vi "Autonomous Independent.vi"   [LabVIEW 2017]
doc: "This VI is called when autonomous begins, and will automatically be terminated when autonomous ends. You can carry out timed or sensor driven robot movement independently without needing to return to the caller."
uses:
  AutonActions.ctl
  WristPositions.ctl
  fec7e146-7db9-40ed-95e9-9a867f74a6f6.vi
  cf8db7aa-b0ae-4ba0-9a67-042f718c3c26.vi
  <vilib>/Rock Robotics/Network Tables/NT Write String.vi
types:
  T1 = cluster{"TrgtCounts":i32, "CurrCounts":dbl, "SlowRng":dbl}
  T2 = cluster{"Heading":dbl, "Target":dbl, "Range":dbl, "GyroSens":dbl}
  T3 = typedef "AutonActions.ctl" = enum16{"Initialize", "Stop", "StraightForward", "StraightBack", "SolenoidControl", "StraightForwardTime", "Release", "Shoot", "Wrist", "GripperToggle", "ElevUp", "ElevDown", "Pause", "ShifterToggle", "", "CubeCollect", "Intake", "ForwardPivot", "BackPivot", "GeneralTurn"}
  T4 = typedef "WristPositions.ctl" = enum16{"AllDown", "AllUp"}
  T5 = cluster{"Action":T3, "DriveEncCnts":i32, "Accel?":bool, "Decel?":bool, "ElevEncCnts":i32, "Action2":T3, "Action2Trigger":i32, "WristPositions":T4, "SlowRng":dbl, "TimeOut":dbl, "GyroSens":dbl, "DriveHeading":dbl}[]
  T6 = cluster{"Action":T3, "DriveEncCnts":i32, "Accel?":bool, "Decel?":bool, "ElevEncCnts":i32, "Action2":T3, "Action2Trigger":i32, "WristPositions":T4, "SlowRng":dbl, "TimeOut":dbl, "GyroSens":dbl, "DriveHeading":dbl}
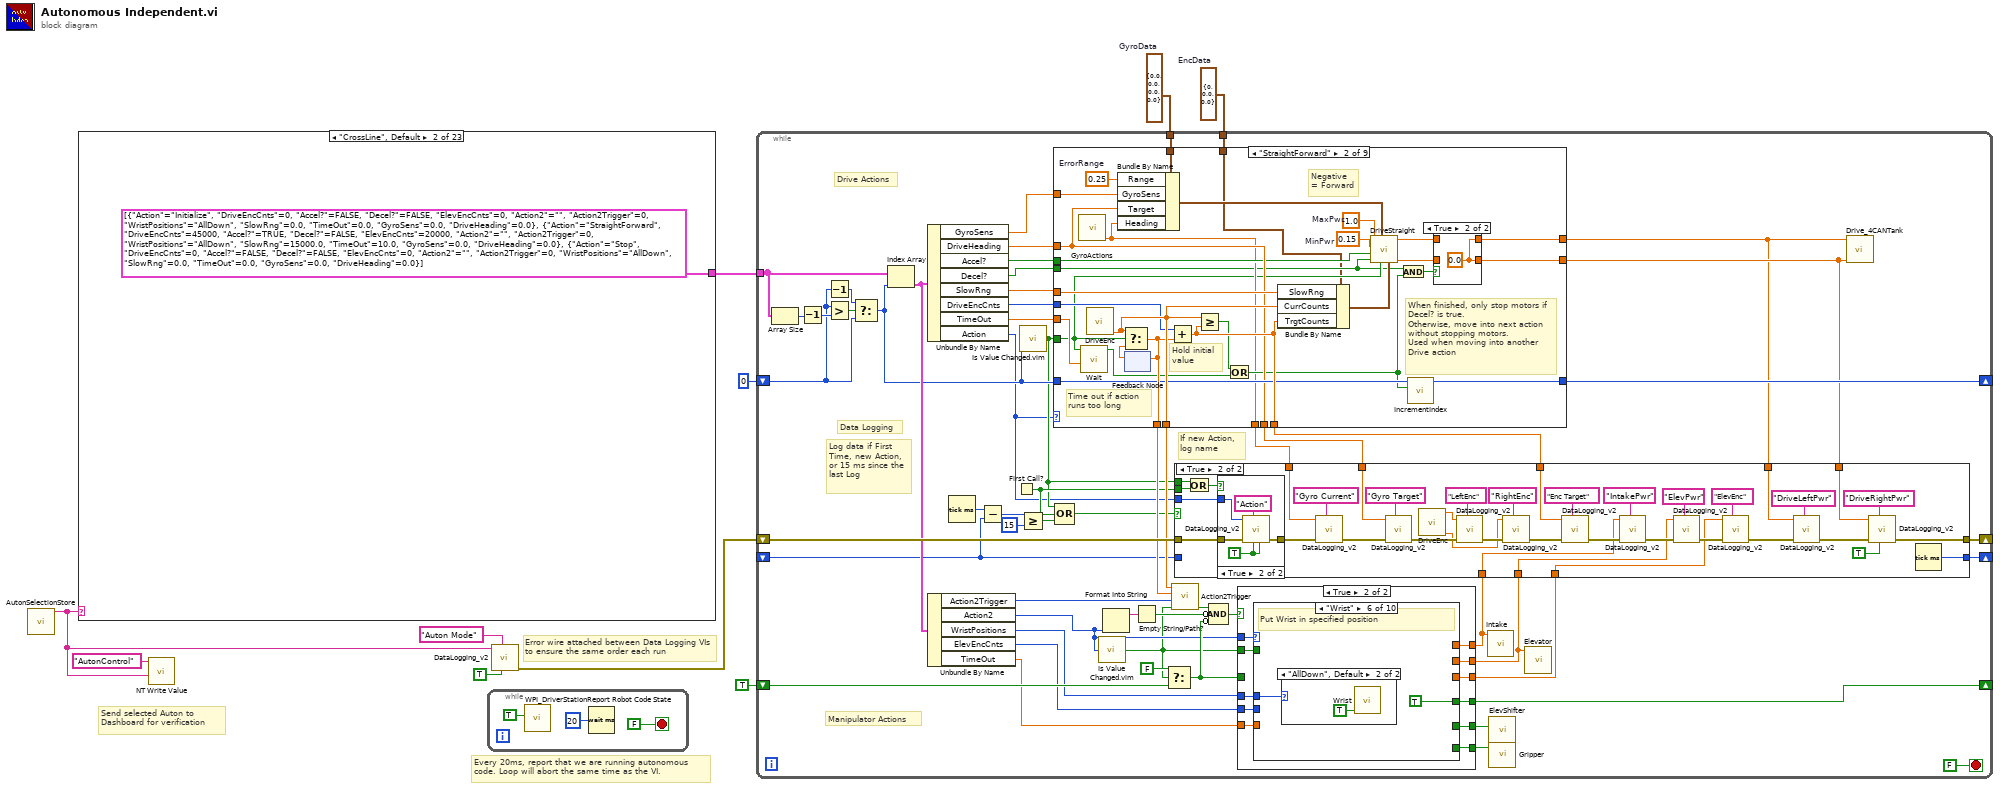
[diagram p0: block diagram]
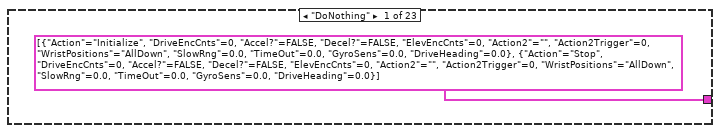
[diagram p2: hidden frame]
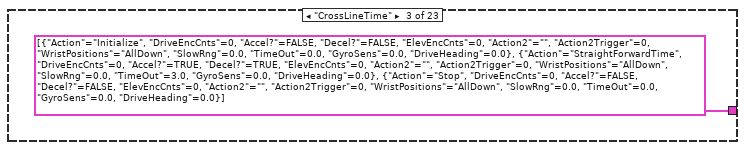
[diagram p3: hidden frame]
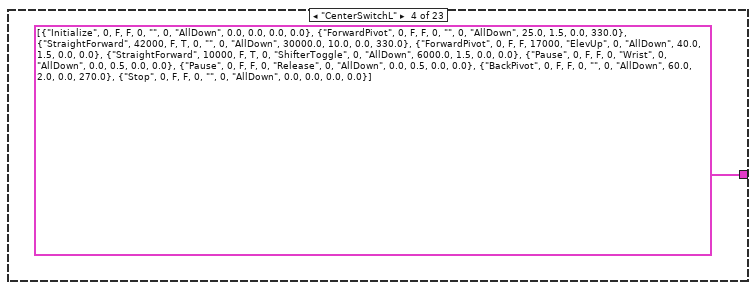
[diagram p4: hidden frame]
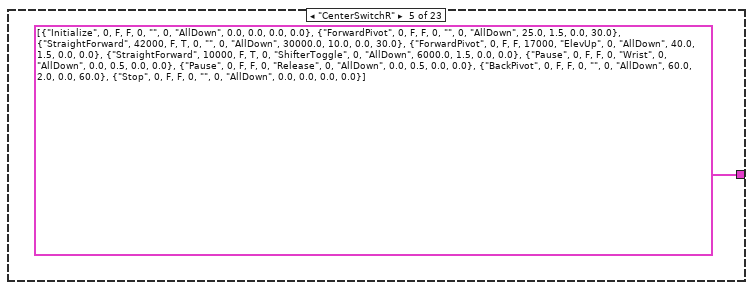
[diagram p5: hidden frame]
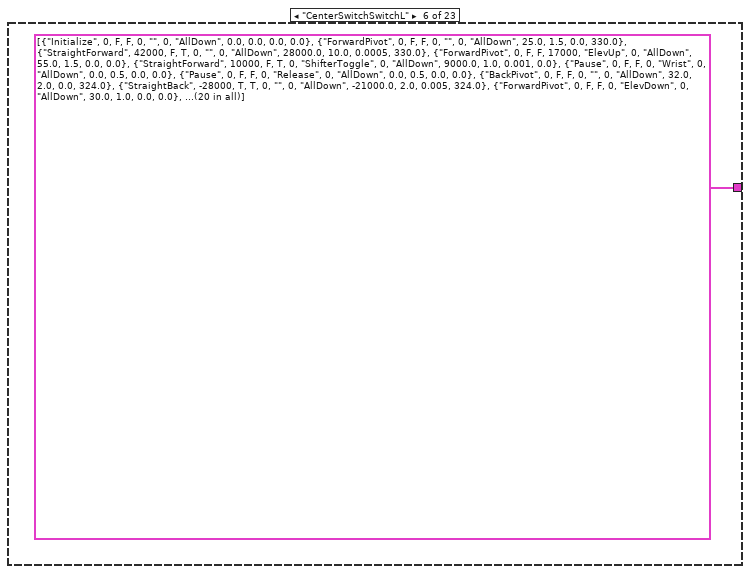
[diagram p6: hidden frame]
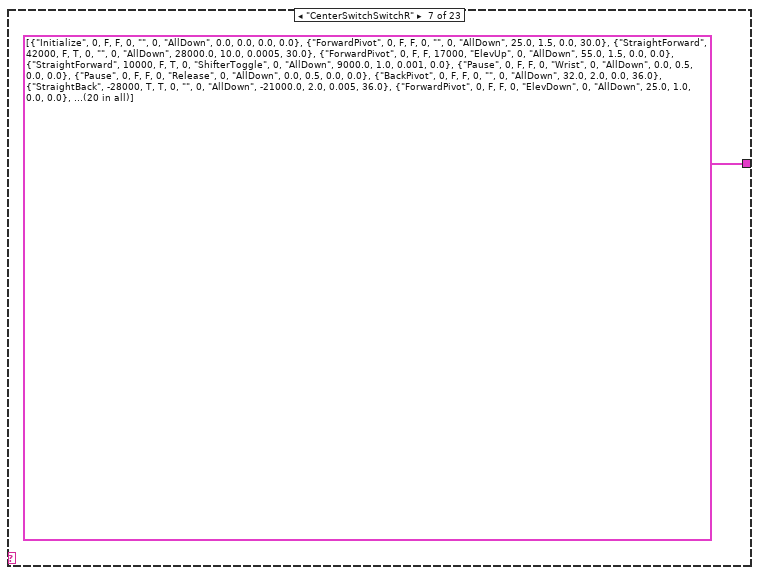
[diagram p7: hidden frame]
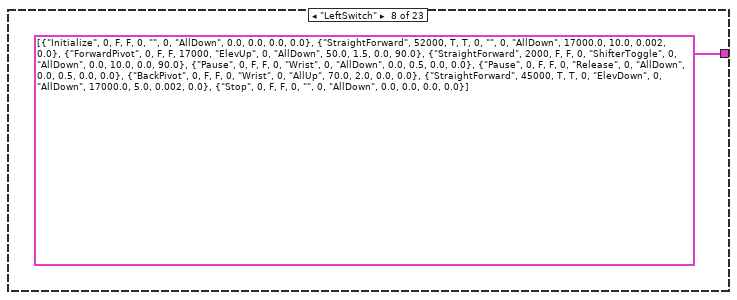
[diagram p8: hidden frame]
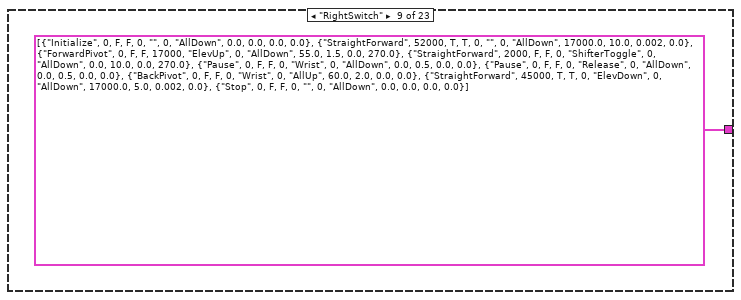
[diagram p9: hidden frame]
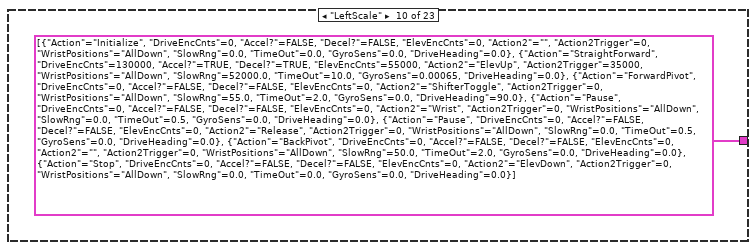
[diagram p10: hidden frame]
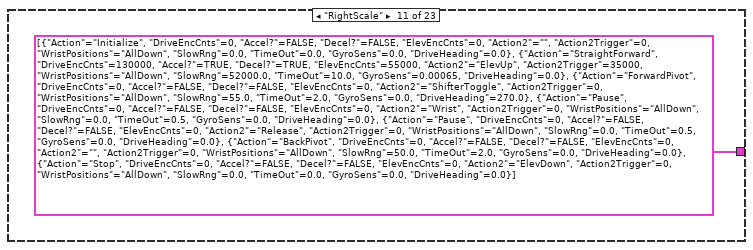
[diagram p11: hidden frame]
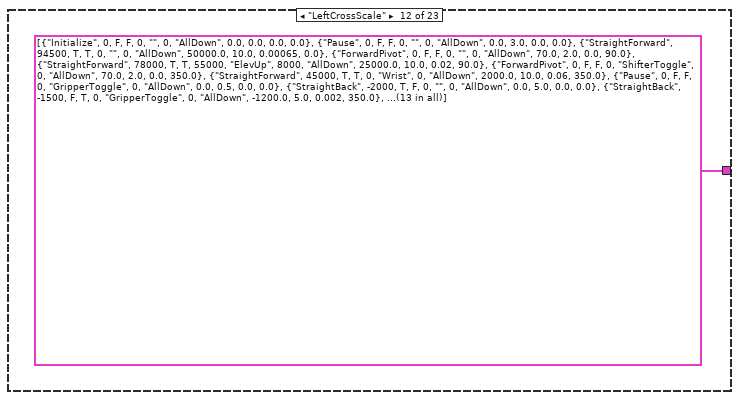
[diagram p12: hidden frame]
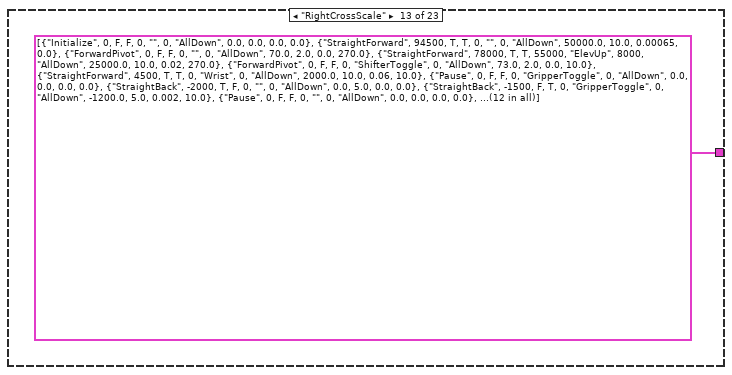
[diagram p13: hidden frame]
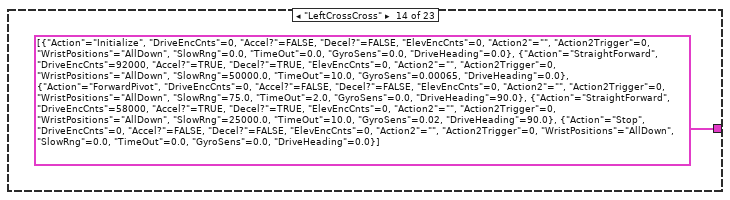
[diagram p14: hidden frame]
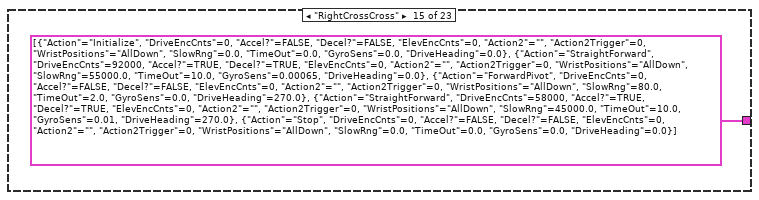
[diagram p15: hidden frame]
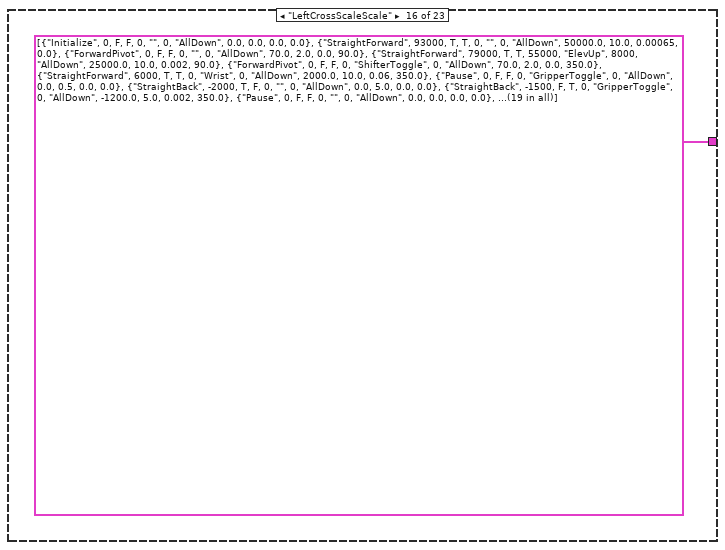
[diagram p16: hidden frame]
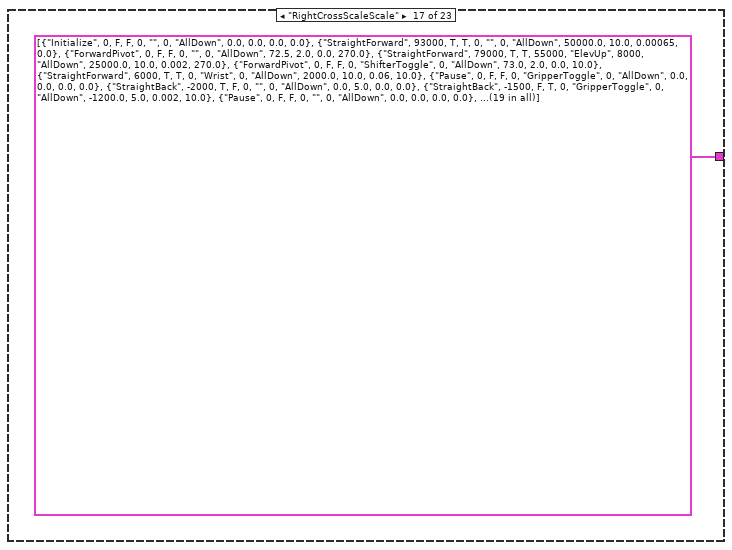
[diagram p17: hidden frame]
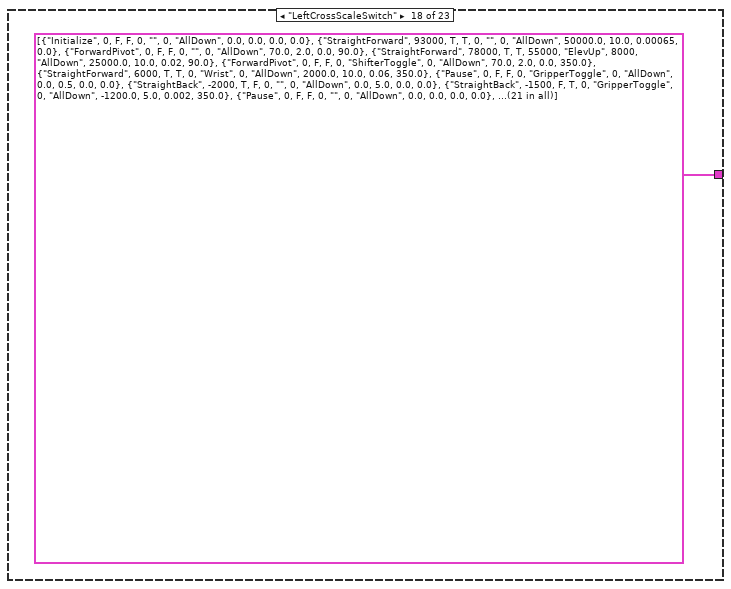
[diagram p18: hidden frame]
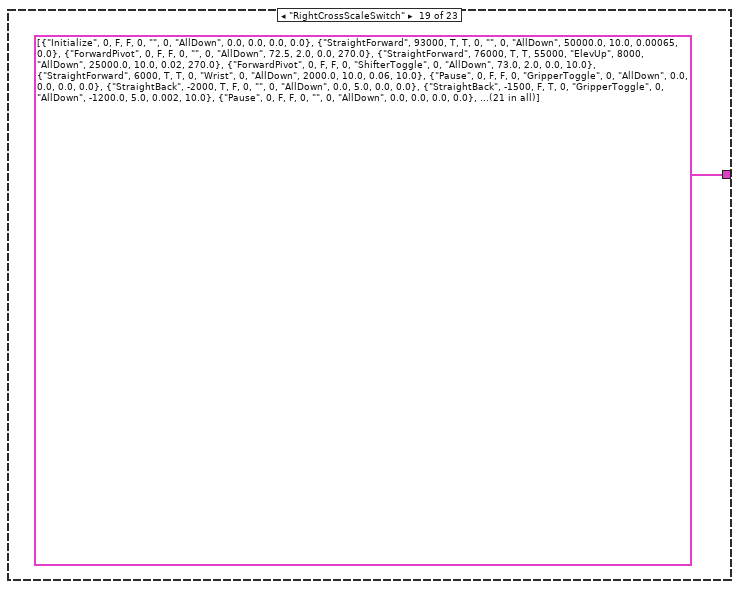
[diagram p19: hidden frame]
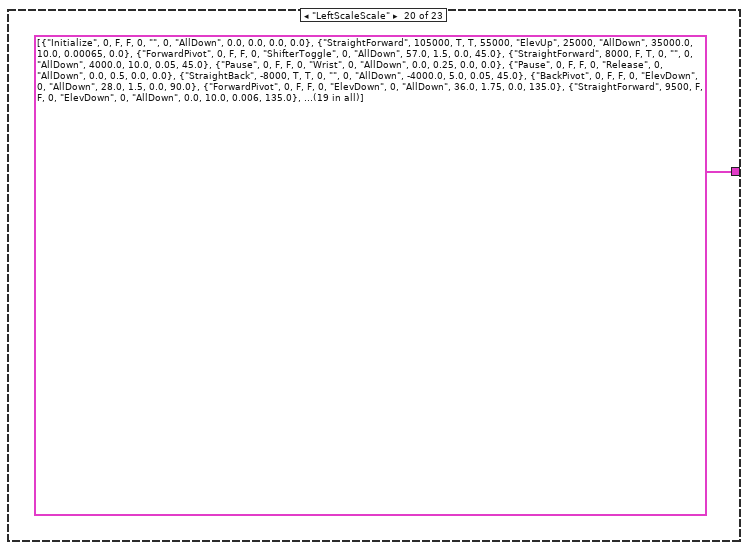
[diagram p20: hidden frame]
diagram:
  w7 = T1 {"TrgtCounts"=0, "CurrCounts"=0.0, "SlowRng"=0.0}  # EncData
  w8 = T2 {"Heading"=0.0, "Target"=0.0, "Range"=0.0, "GyroSens"=0.0}  # GyroData
  # "Error wire attached between Data Logging VIs to ensure the same order each run"
  # "Send selected Auton to Dashboard for verification"
  # "Every 20ms, report that we are running autonomous\ncode. Loop will abort the same time as the VI."
  n1 = call "AutonSelectionStore.vi"() -> ("AutonSelectionOut"=w4:string)  [unwired: 11 in]
  n2 = case shown="\"CrossLine\", Default" w4 {
    tunnel: [T5 [{"Action"=enum."Initialize", "DriveEncCnts"=0, "Accel?"=FALSE, "Decel?"=FALSE, "ElevEncCnts"=0, "Action2"=enum."", "Action2Trigger"=0, "WristPositions"=enum."AllDown", "SlowRng"=0.0, "TimeOut"=0.0, "GyroSens"=0.0, "DriveHeading"=0.0}, {"Action"=enum."Stop", "DriveEncCnts"=0, "Accel?"=FALSE, "Decel?"=FALSE, "ElevEncCnts"=0, "Action2"=enum."", "Action2Trigger"=0, "WristPositions"=enum."AllDown", "SlowRng"=0.0, "TimeOut"=0.0, "GyroSens"=0.0, "DriveHeading"=0.0}] T5 [{"Action"=enum."Initialize", "DriveEncCnts"=0, "Accel?"=FALSE, "Decel?"=FALSE, "ElevEncCnts"=0, "Action2"=enum."", "Action2Trigger"=0, "WristPositions"=enum."AllDown", "SlowRng"=0.0, "TimeOut"=0.0, "GyroSens"=0.0, "DriveHeading"=0.0}, {"Action"=enum."StraightForward", "DriveEncCnts"=45000, "Accel?"=TRUE, "Decel?"=FALSE, "ElevEncCnts"=20000, "Action2"=enum."", "Action2Trigger"=0, "WristPositions"=enum."AllDown", "SlowRng"=15000.0, "TimeOut"=10.0, "GyroSens"=0.0, "DriveHeading"=0.0}, {"Action"=enum."Stop", "DriveEncCnts"=0, "Accel?"=FALSE, "Decel?"=FALSE, "ElevEncCnts"=0, "Action2"=enum."", "Action2Trigger"=0, "WristPositions"=enum."AllDown", "SlowRng"=0.0, "TimeOut"=0.0, "GyroSens"=0.0, "DriveHeading"=0.0}] T5 [{"Action"=enum."Initialize", "DriveEncCnts"=0, "Accel?"=FALSE, "Decel?"=FALSE, "ElevEncCnts"=0, "Action2"=enum."", "Action2Trigger"=0, "WristPositions"=enum."AllDown", "SlowRng"=0.0, "TimeOut"=0.0, "GyroSens"=0.0, "DriveHeading"=0.0}, {"Action"=enum."StraightForwardTime", "DriveEncCnts"=0, "Accel?"=TRUE, "Decel?"=TRUE, "ElevEncCnts"=0, "Action2"=enum."", "Action2Trigger"=0, "WristPositions"=enum."AllDown", "SlowRng"=0.0, "TimeOut"=3.0, "GyroSens"=0.0, "DriveHeading"=0.0}, {"Action"=enum."Stop", "DriveEncCnts"=0, "Accel?"=FALSE, "Decel?"=FALSE, "ElevEncCnts"=0, "Action2"=enum."", "Action2Trigger"=0, "WristPositions"=enum."AllDown", "SlowRng"=0.0, "TimeOut"=0.0, "GyroSens"=0.0, "DriveHeading"=0.0}] T5 [{"Action"=enum."Initialize", "DriveEncCnts"=0, "Accel?"=FALSE, "Decel?"=FALSE, "ElevEncCnts"=0, "Action2"=enum."", "Action2Trigger"=0, "WristPositions"=enum."AllDown", "SlowRng"=0.0, "TimeOut"=0.0, "GyroSens"=0.0, "DriveHeading"=0.0}, {"Action"=enum."ForwardPivot", "DriveEncCnts"=0, "Accel?"=FALSE, "Decel?"=FALSE, "ElevEncCnts"=0, "Action2"=enum."", "Action2Trigger"=0, "WristPositions"=enum."AllDown", "SlowRng"=25.0, "TimeOut"=1.5, "GyroSens"=0.0, "DriveHeading"=330.0}, {"Action"=enum."StraightForward", "DriveEncCnts"=42000, "Accel?"=FALSE, "Decel?"=TRUE, "ElevEncCnts"=0, "Action2"=enum."", "Action2Trigger"=0, "WristPositions"=enum."AllDown", "SlowRng"=30000.0, "TimeOut"=10.0, "GyroSens"=0.0, "DriveHeading"=330.0}, {"Action"=enum."ForwardPivot", "DriveEncCnts"=0, "Accel?"=FALSE, "Decel?"=FALSE, "ElevEncCnts"=17000, "Action2"=enum."ElevUp", "Action2Trigger"=0, "WristPositions"=enum."AllDown", "SlowRng"=40.0, "TimeOut"=1.5, "GyroSens"=0.0, "DriveHeading"=0.0}, {"Action"=enum."StraightForward", "DriveEncCnts"=10000, "Accel?"=FALSE, "Decel?"=TRUE, "ElevEncCnts"=0, "Action2"=enum."ShifterToggle", "Action2Trigger"=0, "WristPositions"=enum."AllDown", "SlowRng"=6000.0, "TimeOut"=1.5, "GyroSens"=0.0, "DriveHeading"=0.0}, {"Action"=enum."Pause", "DriveEncCnts"=0, "Accel?"=FALSE, "Decel?"=FALSE, "ElevEncCnts"=0, "Action2"=enum."Wrist", "Action2Trigger"=0, "WristPositions"=enum."AllDown", "SlowRng"=0.0, "TimeOut"=0.5, "GyroSens"=0.0, "DriveHeading"=0.0}, {"Action"=enum."Pause", "DriveEncCnts"=0, "Accel?"=FALSE, "Decel?"=FALSE, "ElevEncCnts"=0, "Action2"=enum."Release", "Action2Trigger"=0, "WristPositions"=enum."AllDown", "SlowRng"=0.0, "TimeOut"=0.5, "GyroSens"=0.0, "DriveHeading"=0.0}, {"Action"=enum."BackPivot", "DriveEncCnts"=0, "Accel?"=FALSE, "Decel?"=FALSE, "ElevEncCnts"=0, "Action2"=enum."", "Action2Trigger"=0, "WristPositions"=enum."AllDown", "SlowRng"=60.0, "TimeOut"=2.0, "GyroSens"=0.0, "DriveHeading"=270.0}, {"Action"=enum."Stop", "DriveEncCnts"=0, "Accel?"=FALSE, "Decel?"=FALSE, "ElevEncCnts"=0, "Action2"=enum."", "Action2Trigger"=0, "WristPositions"=enum."AllDown", "SlowRng"=0.0, "TimeOut"=0.0, "GyroSens"=0.0, "DriveHeading"=0.0}] T5 [{"Action"=enum."Initialize", "DriveEncCnts"=0, "Accel?"=FALSE, "Decel?"=FALSE, "ElevEncCnts"=0, "Action2"=enum."", "Action2Trigger"=0, "WristPositions"=enum."AllDown", "SlowRng"=0.0, "TimeOut"=0.0, "GyroSens"=0.0, "DriveHeading"=0.0}, {"Action"=enum."ForwardPivot", "DriveEncCnts"=0, "Accel?"=FALSE, "Decel?"=FALSE, "ElevEncCnts"=0, "Action2"=enum."", "Action2Trigger"=0, "WristPositions"=enum."AllDown", "SlowRng"=25.0, "TimeOut"=1.5, "GyroSens"=0.0, "DriveHeading"=30.0}, {"Action"=enum."StraightForward", "DriveEncCnts"=42000, "Accel?"=FALSE, "Decel?"=TRUE, "ElevEncCnts"=0, "Action2"=enum."", "Action2Trigger"=0, "WristPositions"=enum."AllDown", "SlowRng"=30000.0, "TimeOut"=10.0, "GyroSens"=0.0, "DriveHeading"=30.0}, {"Action"=enum."ForwardPivot", "DriveEncCnts"=0, "Accel?"=FALSE, "Decel?"=FALSE, "ElevEncCnts"=17000, "Action2"=enum."ElevUp", "Action2Trigger"=0, "WristPositions"=enum."AllDown", "SlowRng"=40.0, "TimeOut"=1.5, "GyroSens"=0.0, "DriveHeading"=0.0}, {"Action"=enum."StraightForward", "DriveEncCnts"=10000, "Accel?"=FALSE, "Decel?"=TRUE, "ElevEncCnts"=0, "Action2"=enum."ShifterToggle", "Action2Trigger"=0, "WristPositions"=enum."AllDown", "SlowRng"=6000.0, "TimeOut"=1.5, "GyroSens"=0.0, "DriveHeading"=0.0}, {"Action"=enum."Pause", "DriveEncCnts"=0, "Accel?"=FALSE, "Decel?"=FALSE, "ElevEncCnts"=0, "Action2"=enum."Wrist", "Action2Trigger"=0, "WristPositions"=enum."AllDown", "SlowRng"=0.0, "TimeOut"=0.5, "GyroSens"=0.0, "DriveHeading"=0.0}, {"Action"=enum."Pause", "DriveEncCnts"=0, "Accel?"=FALSE, "Decel?"=FALSE, "ElevEncCnts"=0, "Action2"=enum."Release", "Action2Trigger"=0, "WristPositions"=enum."AllDown", "SlowRng"=0.0, "TimeOut"=0.5, "GyroSens"=0.0, "DriveHeading"=0.0}, {"Action"=enum."BackPivot", "DriveEncCnts"=0, "Accel?"=FALSE, "Decel?"=FALSE, "ElevEncCnts"=0, "Action2"=enum."", "Action2Trigger"=0, "WristPositions"=enum."AllDown", "SlowRng"=60.0, "TimeOut"=2.0, "GyroSens"=0.0, "DriveHeading"=60.0}, {"Action"=enum."Stop", "DriveEncCnts"=0, "Accel?"=FALSE, "Decel?"=FALSE, "ElevEncCnts"=0, "Action2"=enum."", "Action2Trigger"=0, "WristPositions"=enum."AllDown", "SlowRng"=0.0, "TimeOut"=0.0, "GyroSens"=0.0, "DriveHeading"=0.0}] T5 [{"Action"=enum."Initialize", "DriveEncCnts"=0, "Accel?"=FALSE, "Decel?"=FALSE, "ElevEncCnts"=0, "Action2"=enum."", "Action2Trigger"=0, "WristPositions"=enum."AllDown", "SlowRng"=0.0, "TimeOut"=0.0, "GyroSens"=0.0, "DriveHeading"=0.0}, {"Action"=enum."ForwardPivot", "DriveEncCnts"=0, "Accel?"=FALSE, "Decel?"=FALSE, "ElevEncCnts"=0, "Action2"=enum."", "Action2Trigger"=0, "WristPositions"=enum."AllDown", "SlowRng"=25.0, "TimeOut"=1.5, "GyroSens"=0.0, "DriveHeading"=330.0}, {"Action"=enum."StraightForward", "DriveEncCnts"=42000, "Accel?"=FALSE, "Decel?"=TRUE, "ElevEncCnts"=0, "Action2"=enum."", "Action2Trigger"=0, "WristPositions"=enum."AllDown", "SlowRng"=28000.0, "TimeOut"=10.0, "GyroSens"=0.0005, "DriveHeading"=330.0}, {"Action"=enum."ForwardPivot", "DriveEncCnts"=0, "Accel?"=FALSE, "Decel?"=FALSE, "ElevEncCnts"=17000, "Action2"=enum."ElevUp", "Action2Trigger"=0, "WristPositions"=enum."AllDown", "SlowRng"=55.0, "TimeOut"=1.5, "GyroSens"=0.0, "DriveHeading"=0.0}, {"Action"=enum."StraightForward", "DriveEncCnts"=10000, "Accel?"=FALSE, "Decel?"=TRUE, "ElevEncCnts"=0, "Action2"=enum."ShifterToggle", "Action2Trigger"=0, "WristPositions"=enum."AllDown", "SlowRng"=9000.0, "TimeOut"=1.0, "GyroSens"=0.001, "DriveHeading"=0.0}, {"Action"=enum."Pause", "DriveEncCnts"=0, "Accel?"=FALSE, "Decel?"=FALSE, "ElevEncCnts"=0, "Action2"=enum."Wrist", "Action2Trigger"=0, "WristPositions"=enum."AllDown", "SlowRng"=0.0, "TimeOut"=0.5, "GyroSens"=0.0, "DriveHeading"=0.0}, {"Action"=enum."Pause", "DriveEncCnts"=0, "Accel?"=FALSE, "Decel?"=FALSE, "ElevEncCnts"=0, "Action2"=enum."Release", "Action2Trigger"=0, "WristPositions"=enum."AllDown", "SlowRng"=0.0, "TimeOut"=0.5, "GyroSens"=0.0, "DriveHeading"=0.0}, {"Action"=enum."BackPivot", "DriveEncCnts"=0, "Accel?"=FALSE, "Decel?"=FALSE, "ElevEncCnts"=0, "Action2"=enum."", "Action2Trigger"=0, "WristPositions"=enum."AllDown", "SlowRng"=32.0, "TimeOut"=2.0, "GyroSens"=0.0, "DriveHeading"=324.0}, {"Action"=enum."StraightBack", "DriveEncCnts"=-28000, "Accel?"=TRUE, "Decel?"=TRUE, "ElevEncCnts"=0, "Action2"=enum."", "Action2Trigger"=0, "WristPositions"=enum."AllDown", "SlowRng"=-21000.0, "TimeOut"=2.0, "GyroSens"=0.005, "DriveHeading"=324.0}, {"Action"=enum."ForwardPivot", "DriveEncCnts"=0, "Accel?"=FALSE, "Decel?"=FALSE, "ElevEncCnts"=0, "Action2"=enum."ElevDown", "Action2Trigger"=0, "WristPositions"=enum."AllDown", "SlowRng"=30.0, "TimeOut"=1.0, "GyroSens"=0.0, "DriveHeading"=0.0}, {"Action"=enum."StraightForward", "DriveEncCnts"=12000, "Accel?"=FALSE, "Decel?"=TRUE, "ElevEncCnts"=0, "Action2"=enum."Intake", "Action2Trigger"=0, "WristPositions"=enum."AllDown", "SlowRng"=6000.0, "TimeOut"=2.0, "GyroSens"=0.003, "DriveHeading"=0.0}, {"Action"=enum."Pause", "DriveEncCnts"=0, "Accel?"=FALSE, "Decel?"=FALSE, "ElevEncCnts"=0, "Action2"=enum."CubeCollect", "Action2Trigger"=0, "WristPositions"=enum."AllDown", "SlowRng"=0.0, "TimeOut"=0.5, "GyroSens"=0.0, "DriveHeading"=0.0}, {"Action"=enum."BackPivot", "DriveEncCnts"=0, "Accel?"=FALSE, "Decel?"=FALSE, "ElevEncCnts"=0, "Action2"=enum."Intake", "Action2Trigger"=0, "WristPositions"=enum."AllDown", "SlowRng"=35.0, "TimeOut"=3.0, "GyroSens"=0.0, "DriveHeading"=310.0}, {"Action"=enum."StraightForward", "DriveEncCnts"=25000, "Accel?"=TRUE, "Decel?"=TRUE, "ElevEncCnts"=17000, "Action2"=enum."ElevUp", "Action2Trigger"=0, "WristPositions"=enum."AllDown", "SlowRng"=16000.0, "TimeOut"=2.0, "GyroSens"=0.0, "DriveHeading"=310.0}, {"Action"=enum."ForwardPivot", "DriveEncCnts"=0, "Accel?"=FALSE, "Decel?"=FALSE, "ElevEncCnts"=0, "Action2"=enum."ShifterToggle", "Action2Trigger"=0, "WristPositions"=enum."AllDown", "SlowRng"=35.0, "TimeOut"=0.75, "GyroSens"=0.0, "DriveHeading"=0.0}, {"Action"=enum."Pause", "DriveEncCnts"=0, "Accel?"=FALSE, "Decel?"=FALSE, "ElevEncCnts"=0, "Action2"=enum."Wrist", "Action2Trigger"=0, "WristPositions"=enum."AllDown", "SlowRng"=0.0, "TimeOut"=0.5, "GyroSens"=0.0, "DriveHeading"=0.0}, {"Action"=enum."Pause", "DriveEncCnts"=0, "Accel?"=FALSE, "Decel?"=FALSE, "ElevEncCnts"=0, "Action2"=enum."Release", "Action2Trigger"=0, "WristPositions"=enum."AllDown", "SlowRng"=0.0, "TimeOut"=0.5, "GyroSens"=0.0, "DriveHeading"=0.0}, {"Action"=enum."StraightBack", "DriveEncCnts"=-10000, "Accel?"=TRUE, "Decel?"=TRUE, "ElevEncCnts"=0, "Action2"=enum."", "Action2Trigger"=0, "WristPositions"=enum."AllDown", "SlowRng"=-7000.0, "TimeOut"=2.5, "GyroSens"=0.0, "DriveHeading"=0.0}, {"Action"=enum."BackPivot", "DriveEncCnts"=0, "Accel?"=FALSE, "Decel?"=FALSE, "ElevEncCnts"=0, "Action2"=enum."ElevDown", "Action2Trigger"=0, "WristPositions"=enum."AllDown", "SlowRng"=55.0, "TimeOut"=1.0, "GyroSens"=0.0, "DriveHeading"=270.0}, {"Action"=enum."Stop", "DriveEncCnts"=0, "Accel?"=FALSE, "Decel?"=FALSE, "ElevEncCnts"=0, "Action2"=enum."ElevDown", "Action2Trigger"=0, "WristPositions"=enum."AllDown", "SlowRng"=0.0, "TimeOut"=0.0, "GyroSens"=0.0, "DriveHeading"=0.0}] T5 [{"Action"=enum."Initialize", "DriveEncCnts"=0, "Accel?"=FALSE, "Decel?"=FALSE, "ElevEncCnts"=0, "Action2"=enum."", "Action2Trigger"=0, "WristPositions"=enum."AllDown", "SlowRng"=0.0, "TimeOut"=0.0, "GyroSens"=0.0, "DriveHeading"=0.0}, {"Action"=enum."ForwardPivot", "DriveEncCnts"=0, "Accel?"=FALSE, "Decel?"=FALSE, "ElevEncCnts"=0, "Action2"=enum."", "Action2Trigger"=0, "WristPositions"=enum."AllDown", "SlowRng"=25.0, "TimeOut"=1.5, "GyroSens"=0.0, "DriveHeading"=30.0}, {"Action"=enum."StraightForward", "DriveEncCnts"=42000, "Accel?"=FALSE, "Decel?"=TRUE, "ElevEncCnts"=0, "Action2"=enum."", "Action2Trigger"=0, "WristPositions"=enum."AllDown", "SlowRng"=28000.0, "TimeOut"=10.0, "GyroSens"=0.0005, "DriveHeading"=30.0}, {"Action"=enum."ForwardPivot", "DriveEncCnts"=0, "Accel?"=FALSE, "Decel?"=FALSE, "ElevEncCnts"=17000, "Action2"=enum."ElevUp", "Action2Trigger"=0, "WristPositions"=enum."AllDown", "SlowRng"=55.0, "TimeOut"=1.5, "GyroSens"=0.0, "DriveHeading"=0.0}, {"Action"=enum."StraightForward", "DriveEncCnts"=10000, "Accel?"=FALSE, "Decel?"=TRUE, "ElevEncCnts"=0, "Action2"=enum."ShifterToggle", "Action2Trigger"=0, "WristPositions"=enum."AllDown", "SlowRng"=9000.0, "TimeOut"=1.0, "GyroSens"=0.001, "DriveHeading"=0.0}, {"Action"=enum."Pause", "DriveEncCnts"=0, "Accel?"=FALSE, "Decel?"=FALSE, "ElevEncCnts"=0, "Action2"=enum."Wrist", "Action2Trigger"=0, "WristPositions"=enum."AllDown", "SlowRng"=0.0, "TimeOut"=0.5, "GyroSens"=0.0, "DriveHeading"=0.0}, {"Action"=enum."Pause", "DriveEncCnts"=0, "Accel?"=FALSE, "Decel?"=FALSE, "ElevEncCnts"=0, "Action2"=enum."Release", "Action2Trigger"=0, "WristPositions"=enum."AllDown", "SlowRng"=0.0, "TimeOut"=0.5, "GyroSens"=0.0, "DriveHeading"=0.0}, {"Action"=enum."BackPivot", "DriveEncCnts"=0, "Accel?"=FALSE, "Decel?"=FALSE, "ElevEncCnts"=0, "Action2"=enum."", "Action2Trigger"=0, "WristPositions"=enum."AllDown", "SlowRng"=32.0, "TimeOut"=2.0, "GyroSens"=0.0, "DriveHeading"=36.0}, {"Action"=enum."StraightBack", "DriveEncCnts"=-28000, "Accel?"=TRUE, "Decel?"=TRUE, "ElevEncCnts"=0, "Action2"=enum."", "Action2Trigger"=0, "WristPositions"=enum."AllDown", "SlowRng"=-21000.0, "TimeOut"=2.0, "GyroSens"=0.005, "DriveHeading"=36.0}, {"Action"=enum."ForwardPivot", "DriveEncCnts"=0, "Accel?"=FALSE, "Decel?"=FALSE, "ElevEncCnts"=0, "Action2"=enum."ElevDown", "Action2Trigger"=0, "WristPositions"=enum."AllDown", "SlowRng"=25.0, "TimeOut"=1.0, "GyroSens"=0.0, "DriveHeading"=0.0}, {"Action"=enum."StraightForward", "DriveEncCnts"=12000, "Accel?"=FALSE, "Decel?"=TRUE, "ElevEncCnts"=0, "Action2"=enum."Intake", "Action2Trigger"=0, "WristPositions"=enum."AllDown", "SlowRng"=6000.0, "TimeOut"=2.0, "GyroSens"=0.003, "DriveHeading"=0.0}, {"Action"=enum."Pause", "DriveEncCnts"=0, "Accel?"=FALSE, "Decel?"=FALSE, "ElevEncCnts"=0, "Action2"=enum."CubeCollect", "Action2Trigger"=0, "WristPositions"=enum."AllDown", "SlowRng"=0.0, "TimeOut"=0.5, "GyroSens"=0.0, "DriveHeading"=0.0}, {"Action"=enum."BackPivot", "DriveEncCnts"=0, "Accel?"=FALSE, "Decel?"=FALSE, "ElevEncCnts"=0, "Action2"=enum."Intake", "Action2Trigger"=0, "WristPositions"=enum."AllDown", "SlowRng"=30.0, "TimeOut"=3.0, "GyroSens"=0.0, "DriveHeading"=50.0}, {"Action"=enum."StraightForward", "DriveEncCnts"=21000, "Accel?"=TRUE, "Decel?"=TRUE, "ElevEncCnts"=17000, "Action2"=enum."ElevUp", "Action2Trigger"=0, "WristPositions"=enum."AllDown", "SlowRng"=13000.0, "TimeOut"=2.0, "GyroSens"=0.0, "DriveHeading"=50.0}, {"Action"=enum."ForwardPivot", "DriveEncCnts"=0, "Accel?"=FALSE, "Decel?"=FALSE, "ElevEncCnts"=0, "Action2"=enum."ShifterToggle", "Action2Trigger"=0, "WristPositions"=enum."AllDown", "SlowRng"=30.0, "TimeOut"=0.75, "GyroSens"=0.0, "DriveHeading"=0.0}, {"Action"=enum."Pause", "DriveEncCnts"=0, "Accel?"=FALSE, "Decel?"=FALSE, "ElevEncCnts"=0, "Action2"=enum."Wrist", "Action2Trigger"=0, "WristPositions"=enum."AllDown", "SlowRng"=0.0, "TimeOut"=0.5, "GyroSens"=0.0, "DriveHeading"=0.0}, {"Action"=enum."Pause", "DriveEncCnts"=0, "Accel?"=FALSE, "Decel?"=FALSE, "ElevEncCnts"=0, "Action2"=enum."Release", "Action2Trigger"=0, "WristPositions"=enum."AllDown", "SlowRng"=0.0, "TimeOut"=0.5, "GyroSens"=0.0, "DriveHeading"=0.0}, {"Action"=enum."StraightBack", "DriveEncCnts"=-10000, "Accel?"=TRUE, "Decel?"=TRUE, "ElevEncCnts"=0, "Action2"=enum."", "Action2Trigger"=0, "WristPositions"=enum."AllDown", "SlowRng"=-7000.0, "TimeOut"=2.5, "GyroSens"=0.0, "DriveHeading"=0.0}, {"Action"=enum."BackPivot", "DriveEncCnts"=0, "Accel?"=FALSE, "Decel?"=FALSE, "ElevEncCnts"=0, "Action2"=enum."ElevDown", "Action2Trigger"=0, "WristPositions"=enum."AllDown", "SlowRng"=50.0, "TimeOut"=1.0, "GyroSens"=0.0, "DriveHeading"=90.0}, {"Action"=enum."Stop", "DriveEncCnts"=0, "Accel?"=FALSE, "Decel?"=FALSE, "ElevEncCnts"=0, "Action2"=enum."ElevDown", "Action2Trigger"=0, "WristPositions"=enum."AllDown", "SlowRng"=0.0, "TimeOut"=0.0, "GyroSens"=0.0, "DriveHeading"=0.0}] T5 [{"Action"=enum."Initialize", "DriveEncCnts"=0, "Accel?"=FALSE, "Decel?"=FALSE, "ElevEncCnts"=0, "Action2"=enum."", "Action2Trigger"=0, "WristPositions"=enum."AllDown", "SlowRng"=0.0, "TimeOut"=0.0, "GyroSens"=0.0, "DriveHeading"=0.0}, {"Action"=enum."StraightForward", "DriveEncCnts"=52000, "Accel?"=TRUE, "Decel?"=TRUE, "ElevEncCnts"=0, "Action2"=enum."", "Action2Trigger"=0, "WristPositions"=enum."AllDown", "SlowRng"=17000.0, "TimeOut"=10.0, "GyroSens"=0.002, "DriveHeading"=0.0}, {"Action"=enum."ForwardPivot", "DriveEncCnts"=0, "Accel?"=FALSE, "Decel?"=FALSE, "ElevEncCnts"=17000, "Action2"=enum."ElevUp", "Action2Trigger"=0, "WristPositions"=enum."AllDown", "SlowRng"=50.0, "TimeOut"=1.5, "GyroSens"=0.0, "DriveHeading"=90.0}, {"Action"=enum."StraightForward", "DriveEncCnts"=2000, "Accel?"=FALSE, "Decel?"=FALSE, "ElevEncCnts"=0, "Action2"=enum."ShifterToggle", "Action2Trigger"=0, "WristPositions"=enum."AllDown", "SlowRng"=0.0, "TimeOut"=10.0, "GyroSens"=0.0, "DriveHeading"=90.0}, {"Action"=enum."Pause", "DriveEncCnts"=0, "Accel?"=FALSE, "Decel?"=FALSE, "ElevEncCnts"=0, "Action2"=enum."Wrist", "Action2Trigger"=0, "WristPositions"=enum."AllDown", "SlowRng"=0.0, "TimeOut"=0.5, "GyroSens"=0.0, "DriveHeading"=0.0}, {"Action"=enum."Pause", "DriveEncCnts"=0, "Accel?"=FALSE, "Decel?"=FALSE, "ElevEncCnts"=0, "Action2"=enum."Release", "Action2Trigger"=0, "WristPositions"=enum."AllDown", "SlowRng"=0.0, "TimeOut"=0.5, "GyroSens"=0.0, "DriveHeading"=0.0}, {"Action"=enum."BackPivot", "DriveEncCnts"=0, "Accel?"=FALSE, "Decel?"=FALSE, "ElevEncCnts"=0, "Action2"=enum."Wrist", "Action2Trigger"=0, "WristPositions"=enum."AllUp", "SlowRng"=70.0, "TimeOut"=2.0, "GyroSens"=0.0, "DriveHeading"=0.0}, {"Action"=enum."StraightForward", "DriveEncCnts"=45000, "Accel?"=TRUE, "Decel?"=TRUE, "ElevEncCnts"=0, "Action2"=enum."ElevDown", "Action2Trigger"=0, "WristPositions"=enum."AllDown", "SlowRng"=17000.0, "TimeOut"=5.0, "GyroSens"=0.002, "DriveHeading"=0.0}, {"Action"=enum."Stop", "DriveEncCnts"=0, "Accel?"=FALSE, "Decel?"=FALSE, "ElevEncCnts"=0, "Action2"=enum."", "Action2Trigger"=0, "WristPositions"=enum."AllDown", "SlowRng"=0.0, "TimeOut"=0.0, "GyroSens"=0.0, "DriveHeading"=0.0}] T5 [{"Action"=enum."Initialize", "DriveEncCnts"=0, "Accel?"=FALSE, "Decel?"=FALSE, "ElevEncCnts"=0, "Action2"=enum."", "Action2Trigger"=0, "WristPositions"=enum."AllDown", "SlowRng"=0.0, "TimeOut"=0.0, "GyroSens"=0.0, "DriveHeading"=0.0}, {"Action"=enum."StraightForward", "DriveEncCnts"=52000, "Accel?"=TRUE, "Decel?"=TRUE, "ElevEncCnts"=0, "Action2"=enum."", "Action2Trigger"=0, "WristPositions"=enum."AllDown", "SlowRng"=17000.0, "TimeOut"=10.0, "GyroSens"=0.002, "DriveHeading"=0.0}, {"Action"=enum."ForwardPivot", "DriveEncCnts"=0, "Accel?"=FALSE, "Decel?"=FALSE, "ElevEncCnts"=17000, "Action2"=enum."ElevUp", "Action2Trigger"=0, "WristPositions"=enum."AllDown", "SlowRng"=55.0, "TimeOut"=1.5, "GyroSens"=0.0, "DriveHeading"=270.0}, {"Action"=enum."StraightForward", "DriveEncCnts"=2000, "Accel?"=FALSE, "Decel?"=FALSE, "ElevEncCnts"=0, "Action2"=enum."ShifterToggle", "Action2Trigger"=0, "WristPositions"=enum."AllDown", "SlowRng"=0.0, "TimeOut"=10.0, "GyroSens"=0.0, "DriveHeading"=270.0}, {"Action"=enum."Pause", "DriveEncCnts"=0, "Accel?"=FALSE, "Decel?"=FALSE, "ElevEncCnts"=0, "Action2"=enum."Wrist", "Action2Trigger"=0, "WristPositions"=enum."AllDown", "SlowRng"=0.0, "TimeOut"=0.5, "GyroSens"=0.0, "DriveHeading"=0.0}, {"Action"=enum."Pause", "DriveEncCnts"=0, "Accel?"=FALSE, "Decel?"=FALSE, "ElevEncCnts"=0, "Action2"=enum."Release", "Action2Trigger"=0, "WristPositions"=enum."AllDown", "SlowRng"=0.0, "TimeOut"=0.5, "GyroSens"=0.0, "DriveHeading"=0.0}, {"Action"=enum."BackPivot", "DriveEncCnts"=0, "Accel?"=FALSE, "Decel?"=FALSE, "ElevEncCnts"=0, "Action2"=enum."Wrist", "Action2Trigger"=0, "WristPositions"=enum."AllUp", "SlowRng"=60.0, "TimeOut"=2.0, "GyroSens"=0.0, "DriveHeading"=0.0}, {"Action"=enum."StraightForward", "DriveEncCnts"=45000, "Accel?"=TRUE, "Decel?"=TRUE, "ElevEncCnts"=0, "Action2"=enum."ElevDown", "Action2Trigger"=0, "WristPositions"=enum."AllDown", "SlowRng"=17000.0, "TimeOut"=5.0, "GyroSens"=0.002, "DriveHeading"=0.0}, {"Action"=enum."Stop", "DriveEncCnts"=0, "Accel?"=FALSE, "Decel?"=FALSE, "ElevEncCnts"=0, "Action2"=enum."", "Action2Trigger"=0, "WristPositions"=enum."AllDown", "SlowRng"=0.0, "TimeOut"=0.0, "GyroSens"=0.0, "DriveHeading"=0.0}] T5 [{"Action"=enum."Initialize", "DriveEncCnts"=0, "Accel?"=FALSE, "Decel?"=FALSE, "ElevEncCnts"=0, "Action2"=enum."", "Action2Trigger"=0, "WristPositions"=enum."AllDown", "SlowRng"=0.0, "TimeOut"=0.0, "GyroSens"=0.0, "DriveHeading"=0.0}, {"Action"=enum."StraightForward", "DriveEncCnts"=130000, "Accel?"=TRUE, "Decel?"=TRUE, "ElevEncCnts"=55000, "Action2"=enum."ElevUp", "Action2Trigger"=35000, "WristPositions"=enum."AllDown", "SlowRng"=52000.0, "TimeOut"=10.0, "GyroSens"=0.00065, "DriveHeading"=0.0}, {"Action"=enum."ForwardPivot", "DriveEncCnts"=0, "Accel?"=FALSE, "Decel?"=FALSE, "ElevEncCnts"=0, "Action2"=enum."ShifterToggle", "Action2Trigger"=0, "WristPositions"=enum."AllDown", "SlowRng"=55.0, "TimeOut"=2.0, "GyroSens"=0.0, "DriveHeading"=90.0}, {"Action"=enum."Pause", "DriveEncCnts"=0, "Accel?"=FALSE, "Decel?"=FALSE, "ElevEncCnts"=0, "Action2"=enum."Wrist", "Action2Trigger"=0, "WristPositions"=enum."AllDown", "SlowRng"=0.0, "TimeOut"=0.5, "GyroSens"=0.0, "DriveHeading"=0.0}, {"Action"=enum."Pause", "DriveEncCnts"=0, "Accel?"=FALSE, "Decel?"=FALSE, "ElevEncCnts"=0, "Action2"=enum."Release", "Action2Trigger"=0, "WristPositions"=enum."AllDown", "SlowRng"=0.0, "TimeOut"=0.5, "GyroSens"=0.0, "DriveHeading"=0.0}, {"Action"=enum."BackPivot", "DriveEncCnts"=0, "Accel?"=FALSE, "Decel?"=FALSE, "ElevEncCnts"=0, "Action2"=enum."", "Action2Trigger"=0, "WristPositions"=enum."AllDown", "SlowRng"=50.0, "TimeOut"=2.0, "GyroSens"=0.0, "DriveHeading"=0.0}, {"Action"=enum."Stop", "DriveEncCnts"=0, "Accel?"=FALSE, "Decel?"=FALSE, "ElevEncCnts"=0, "Action2"=enum."ElevDown", "Action2Trigger"=0, "WristPositions"=enum."AllDown", "SlowRng"=0.0, "TimeOut"=0.0, "GyroSens"=0.0, "DriveHeading"=0.0}] T5 [{"Action"=enum."Initialize", "DriveEncCnts"=0, "Accel?"=FALSE, "Decel?"=FALSE, "ElevEncCnts"=0, "Action2"=enum."", "Action2Trigger"=0, "WristPositions"=enum."AllDown", "SlowRng"=0.0, "TimeOut"=0.0, "GyroSens"=0.0, "DriveHeading"=0.0}, {"Action"=enum."StraightForward", "DriveEncCnts"=130000, "Accel?"=TRUE, "Decel?"=TRUE, "ElevEncCnts"=55000, "Action2"=enum."ElevUp", "Action2Trigger"=35000, "WristPositions"=enum."AllDown", "SlowRng"=52000.0, "TimeOut"=10.0, "GyroSens"=0.00065, "DriveHeading"=0.0}, {"Action"=enum."ForwardPivot", "DriveEncCnts"=0, "Accel?"=FALSE, "Decel?"=FALSE, "ElevEncCnts"=0, "Action2"=enum."ShifterToggle", "Action2Trigger"=0, "WristPositions"=enum."AllDown", "SlowRng"=55.0, "TimeOut"=2.0, "GyroSens"=0.0, "DriveHeading"=270.0}, {"Action"=enum."Pause", "DriveEncCnts"=0, "Accel?"=FALSE, "Decel?"=FALSE, "ElevEncCnts"=0, "Action2"=enum."Wrist", "Action2Trigger"=0, "WristPositions"=enum."AllDown", "SlowRng"=0.0, "TimeOut"=0.5, "GyroSens"=0.0, "DriveHeading"=0.0}, {"Action"=enum."Pause", "DriveEncCnts"=0, "Accel?"=FALSE, "Decel?"=FALSE, "ElevEncCnts"=0, "Action2"=enum."Release", "Action2Trigger"=0, "WristPositions"=enum."AllDown", "SlowRng"=0.0, "TimeOut"=0.5, "GyroSens"=0.0, "DriveHeading"=0.0}, {"Action"=enum."BackPivot", "DriveEncCnts"=0, "Accel?"=FALSE, "Decel?"=FALSE, "ElevEncCnts"=0, "Action2"=enum."", "Action2Trigger"=0, "WristPositions"=enum."AllDown", "SlowRng"=50.0, "TimeOut"=2.0, "GyroSens"=0.0, "DriveHeading"=0.0}, {"Action"=enum."Stop", "DriveEncCnts"=0, "Accel?"=FALSE, "Decel?"=FALSE, "ElevEncCnts"=0, "Action2"=enum."ElevDown", "Action2Trigger"=0, "WristPositions"=enum."AllDown", "SlowRng"=0.0, "TimeOut"=0.0, "GyroSens"=0.0, "DriveHeading"=0.0}] T5 [{"Action"=enum."Initialize", "DriveEncCnts"=0, "Accel?"=FALSE, "Decel?"=FALSE, "ElevEncCnts"=0, "Action2"=enum."", "Action2Trigger"=0, "WristPositions"=enum."AllDown", "SlowRng"=0.0, "TimeOut"=0.0, "GyroSens"=0.0, "DriveHeading"=0.0}, {"Action"=enum."Pause", "DriveEncCnts"=0, "Accel?"=FALSE, "Decel?"=FALSE, "ElevEncCnts"=0, "Action2"=enum."", "Action2Trigger"=0, "WristPositions"=enum."AllDown", "SlowRng"=0.0, "TimeOut"=3.0, "GyroSens"=0.0, "DriveHeading"=0.0}, {"Action"=enum."StraightForward", "DriveEncCnts"=94500, "Accel?"=TRUE, "Decel?"=TRUE, "ElevEncCnts"=0, "Action2"=enum."", "Action2Trigger"=0, "WristPositions"=enum."AllDown", "SlowRng"=50000.0, "TimeOut"=10.0, "GyroSens"=0.00065, "DriveHeading"=0.0}, {"Action"=enum."ForwardPivot", "DriveEncCnts"=0, "Accel?"=FALSE, "Decel?"=FALSE, "ElevEncCnts"=0, "Action2"=enum."", "Action2Trigger"=0, "WristPositions"=enum."AllDown", "SlowRng"=70.0, "TimeOut"=2.0, "GyroSens"=0.0, "DriveHeading"=90.0}, {"Action"=enum."StraightForward", "DriveEncCnts"=78000, "Accel?"=TRUE, "Decel?"=TRUE, "ElevEncCnts"=55000, "Action2"=enum."ElevUp", "Action2Trigger"=8000, "WristPositions"=enum."AllDown", "SlowRng"=25000.0, "TimeOut"=10.0, "GyroSens"=0.02, "DriveHeading"=90.0}, {"Action"=enum."ForwardPivot", "DriveEncCnts"=0, "Accel?"=FALSE, "Decel?"=FALSE, "ElevEncCnts"=0, "Action2"=enum."ShifterToggle", "Action2Trigger"=0, "WristPositions"=enum."AllDown", "SlowRng"=70.0, "TimeOut"=2.0, "GyroSens"=0.0, "DriveHeading"=350.0}, {"Action"=enum."StraightForward", "DriveEncCnts"=45000, "Accel?"=TRUE, "Decel?"=TRUE, "ElevEncCnts"=0, "Action2"=enum."Wrist", "Action2Trigger"=0, "WristPositions"=enum."AllDown", "SlowRng"=2000.0, "TimeOut"=10.0, "GyroSens"=0.06, "DriveHeading"=350.0}, {"Action"=enum."Pause", "DriveEncCnts"=0, "Accel?"=FALSE, "Decel?"=FALSE, "ElevEncCnts"=0, "Action2"=enum."GripperToggle", "Action2Trigger"=0, "WristPositions"=enum."AllDown", "SlowRng"=0.0, "TimeOut"=0.5, "GyroSens"=0.0, "DriveHeading"=0.0}, {"Action"=enum."StraightBack", "DriveEncCnts"=-2000, "Accel?"=TRUE, "Decel?"=FALSE, "ElevEncCnts"=0, "Action2"=enum."", "Action2Trigger"=0, "WristPositions"=enum."AllDown", "SlowRng"=0.0, "TimeOut"=5.0, "GyroSens"=0.0, "DriveHeading"=0.0}, {"Action"=enum."StraightBack", "DriveEncCnts"=-1500, "Accel?"=FALSE, "Decel?"=TRUE, "ElevEncCnts"=0, "Action2"=enum."GripperToggle", "Action2Trigger"=0, "WristPositions"=enum."AllDown", "SlowRng"=-1200.0, "TimeOut"=5.0, "GyroSens"=0.002, "DriveHeading"=350.0}, {"Action"=enum."Pause", "DriveEncCnts"=0, "Accel?"=FALSE, "Decel?"=FALSE, "ElevEncCnts"=0, "Action2"=enum."", "Action2Trigger"=0, "WristPositions"=enum."AllDown", "SlowRng"=0.0, "TimeOut"=0.0, "GyroSens"=0.0, "DriveHeading"=0.0}, {"Action"=enum."BackPivot", "DriveEncCnts"=0, "Accel?"=FALSE, "Decel?"=FALSE, "ElevEncCnts"=0, "Action2"=enum."ElevDown", "Action2Trigger"=0, "WristPositions"=enum."AllDown", "SlowRng"=60.0, "TimeOut"=2.0, "GyroSens"=0.0, "DriveHeading"=45.0}, {"Action"=enum."Stop", "DriveEncCnts"=0, "Accel?"=FALSE, "Decel?"=FALSE, "ElevEncCnts"=0, "Action2"=enum."", "Action2Trigger"=0, "WristPositions"=enum."AllDown", "SlowRng"=0.0, "TimeOut"=0.0, "GyroSens"=0.0, "DriveHeading"=0.0}] T5 [{"Action"=enum."Initialize", "DriveEncCnts"=0, "Accel?"=FALSE, "Decel?"=FALSE, "ElevEncCnts"=0, "Action2"=enum."", "Action2Trigger"=0, "WristPositions"=enum."AllDown", "SlowRng"=0.0, "TimeOut"=0.0, "GyroSens"=0.0, "DriveHeading"=0.0}, {"Action"=enum."StraightForward", "DriveEncCnts"=94500, "Accel?"=TRUE, "Decel?"=TRUE, "ElevEncCnts"=0, "Action2"=enum."", "Action2Trigger"=0, "WristPositions"=enum."AllDown", "SlowRng"=50000.0, "TimeOut"=10.0, "GyroSens"=0.00065, "DriveHeading"=0.0}, {"Action"=enum."ForwardPivot", "DriveEncCnts"=0, "Accel?"=FALSE, "Decel?"=FALSE, "ElevEncCnts"=0, "Action2"=enum."", "Action2Trigger"=0, "WristPositions"=enum."AllDown", "SlowRng"=70.0, "TimeOut"=2.0, "GyroSens"=0.0, "DriveHeading"=270.0}, {"Action"=enum."StraightForward", "DriveEncCnts"=78000, "Accel?"=TRUE, "Decel?"=TRUE, "ElevEncCnts"=55000, "Action2"=enum."ElevUp", "Action2Trigger"=8000, "WristPositions"=enum."AllDown", "SlowRng"=25000.0, "TimeOut"=10.0, "GyroSens"=0.02, "DriveHeading"=270.0}, {"Action"=enum."ForwardPivot", "DriveEncCnts"=0, "Accel?"=FALSE, "Decel?"=FALSE, "ElevEncCnts"=0, "Action2"=enum."ShifterToggle", "Action2Trigger"=0, "WristPositions"=enum."AllDown", "SlowRng"=73.0, "TimeOut"=2.0, "GyroSens"=0.0, "DriveHeading"=10.0}, {"Action"=enum."StraightForward", "DriveEncCnts"=4500, "Accel?"=TRUE, "Decel?"=TRUE, "ElevEncCnts"=0, "Action2"=enum."Wrist", "Action2Trigger"=0, "WristPositions"=enum."AllDown", "SlowRng"=2000.0, "TimeOut"=10.0, "GyroSens"=0.06, "DriveHeading"=10.0}, {"Action"=enum."Pause", "DriveEncCnts"=0, "Accel?"=FALSE, "Decel?"=FALSE, "ElevEncCnts"=0, "Action2"=enum."GripperToggle", "Action2Trigger"=0, "WristPositions"=enum."AllDown", "SlowRng"=0.0, "TimeOut"=0.0, "GyroSens"=0.0, "DriveHeading"=0.0}, {"Action"=enum."StraightBack", "DriveEncCnts"=-2000, "Accel?"=TRUE, "Decel?"=FALSE, "ElevEncCnts"=0, "Action2"=enum."", "Action2Trigger"=0, "WristPositions"=enum."AllDown", "SlowRng"=0.0, "TimeOut"=5.0, "GyroSens"=0.0, "DriveHeading"=0.0}, {"Action"=enum."StraightBack", "DriveEncCnts"=-1500, "Accel?"=FALSE, "Decel?"=TRUE, "ElevEncCnts"=0, "Action2"=enum."GripperToggle", "Action2Trigger"=0, "WristPositions"=enum."AllDown", "SlowRng"=-1200.0, "TimeOut"=5.0, "GyroSens"=0.002, "DriveHeading"=10.0}, {"Action"=enum."Pause", "DriveEncCnts"=0, "Accel?"=FALSE, "Decel?"=FALSE, "ElevEncCnts"=0, "Action2"=enum."", "Action2Trigger"=0, "WristPositions"=enum."AllDown", "SlowRng"=0.0, "TimeOut"=0.0, "GyroSens"=0.0, "DriveHeading"=0.0}, {"Action"=enum."BackPivot", "DriveEncCnts"=0, "Accel?"=FALSE, "Decel?"=FALSE, "ElevEncCnts"=0, "Action2"=enum."ElevDown", "Action2Trigger"=0, "WristPositions"=enum."AllDown", "SlowRng"=60.0, "TimeOut"=2.0, "GyroSens"=0.0, "DriveHeading"=315.0}, {"Action"=enum."Stop", "DriveEncCnts"=0, "Accel?"=FALSE, "Decel?"=FALSE, "ElevEncCnts"=0, "Action2"=enum."", "Action2Trigger"=0, "WristPositions"=enum."AllDown", "SlowRng"=0.0, "TimeOut"=0.0, "GyroSens"=0.0, "DriveHeading"=0.0}] T5 [{"Action"=enum."Initialize", "DriveEncCnts"=0, "Accel?"=FALSE, "Decel?"=FALSE, "ElevEncCnts"=0, "Action2"=enum."", "Action2Trigger"=0, "WristPositions"=enum."AllDown", "SlowRng"=0.0, "TimeOut"=0.0, "GyroSens"=0.0, "DriveHeading"=0.0}, {"Action"=enum."StraightForward", "DriveEncCnts"=92000, "Accel?"=TRUE, "Decel?"=TRUE, "ElevEncCnts"=0, "Action2"=enum."", "Action2Trigger"=0, "WristPositions"=enum."AllDown", "SlowRng"=50000.0, "TimeOut"=10.0, "GyroSens"=0.00065, "DriveHeading"=0.0}, {"Action"=enum."ForwardPivot", "DriveEncCnts"=0, "Accel?"=FALSE, "Decel?"=FALSE, "ElevEncCnts"=0, "Action2"=enum."", "Action2Trigger"=0, "WristPositions"=enum."AllDown", "SlowRng"=75.0, "TimeOut"=2.0, "GyroSens"=0.0, "DriveHeading"=90.0}, {"Action"=enum."StraightForward", "DriveEncCnts"=58000, "Accel?"=TRUE, "Decel?"=TRUE, "ElevEncCnts"=0, "Action2"=enum."", "Action2Trigger"=0, "WristPositions"=enum."AllDown", "SlowRng"=25000.0, "TimeOut"=10.0, "GyroSens"=0.02, "DriveHeading"=90.0}, {"Action"=enum."Stop", "DriveEncCnts"=0, "Accel?"=FALSE, "Decel?"=FALSE, "ElevEncCnts"=0, "Action2"=enum."", "Action2Trigger"=0, "WristPositions"=enum."AllDown", "SlowRng"=0.0, "TimeOut"=0.0, "GyroSens"=0.0, "DriveHeading"=0.0}] T5 [{"Action"=enum."Initialize", "DriveEncCnts"=0, "Accel?"=FALSE, "Decel?"=FALSE, "ElevEncCnts"=0, "Action2"=enum."", "Action2Trigger"=0, "WristPositions"=enum."AllDown", "SlowRng"=0.0, "TimeOut"=0.0, "GyroSens"=0.0, "DriveHeading"=0.0}, {"Action"=enum."StraightForward", "DriveEncCnts"=92000, "Accel?"=TRUE, "Decel?"=TRUE, "ElevEncCnts"=0, "Action2"=enum."", "Action2Trigger"=0, "WristPositions"=enum."AllDown", "SlowRng"=55000.0, "TimeOut"=10.0, "GyroSens"=0.00065, "DriveHeading"=0.0}, {"Action"=enum."ForwardPivot", "DriveEncCnts"=0, "Accel?"=FALSE, "Decel?"=FALSE, "ElevEncCnts"=0, "Action2"=enum."", "Action2Trigger"=0, "WristPositions"=enum."AllDown", "SlowRng"=80.0, "TimeOut"=2.0, "GyroSens"=0.0, "DriveHeading"=270.0}, {"Action"=enum."StraightForward", "DriveEncCnts"=58000, "Accel?"=TRUE, "Decel?"=TRUE, "ElevEncCnts"=0, "Action2"=enum."", "Action2Trigger"=0, "WristPositions"=enum."AllDown", "SlowRng"=45000.0, "TimeOut"=10.0, "GyroSens"=0.01, "DriveHeading"=270.0}, {"Action"=enum."Stop", "DriveEncCnts"=0, "Accel?"=FALSE, "Decel?"=FALSE, "ElevEncCnts"=0, "Action2"=enum."", "Action2Trigger"=0, "WristPositions"=enum."AllDown", "SlowRng"=0.0, "TimeOut"=0.0, "GyroSens"=0.0, "DriveHeading"=0.0}] T5 [{"Action"=enum."Initialize", "DriveEncCnts"=0, "Accel?"=FALSE, "Decel?"=FALSE, "ElevEncCnts"=0, "Action2"=enum."", "Action2Trigger"=0, "WristPositions"=enum."AllDown", "SlowRng"=0.0, "TimeOut"=0.0, "GyroSens"=0.0, "DriveHeading"=0.0}, {"Action"=enum."StraightForward", "DriveEncCnts"=93000, "Accel?"=TRUE, "Decel?"=TRUE, "ElevEncCnts"=0, "Action2"=enum."", "Action2Trigger"=0, "WristPositions"=enum."AllDown", "SlowRng"=50000.0, "TimeOut"=10.0, "GyroSens"=0.00065, "DriveHeading"=0.0}, {"Action"=enum."ForwardPivot", "DriveEncCnts"=0, "Accel?"=FALSE, "Decel?"=FALSE, "ElevEncCnts"=0, "Action2"=enum."", "Action2Trigger"=0, "WristPositions"=enum."AllDown", "SlowRng"=70.0, "TimeOut"=2.0, "GyroSens"=0.0, "DriveHeading"=90.0}, {"Action"=enum."StraightForward", "DriveEncCnts"=79000, "Accel?"=TRUE, "Decel?"=TRUE, "ElevEncCnts"=55000, "Action2"=enum."ElevUp", "Action2Trigger"=8000, "WristPositions"=enum."AllDown", "SlowRng"=25000.0, "TimeOut"=10.0, "GyroSens"=0.002, "DriveHeading"=90.0}, {"Action"=enum."ForwardPivot", "DriveEncCnts"=0, "Accel?"=FALSE, "Decel?"=FALSE, "ElevEncCnts"=0, "Action2"=enum."ShifterToggle", "Action2Trigger"=0, "WristPositions"=enum."AllDown", "SlowRng"=70.0, "TimeOut"=2.0, "GyroSens"=0.0, "DriveHeading"=350.0}, {"Action"=enum."StraightForward", "DriveEncCnts"=6000, "Accel?"=TRUE, "Decel?"=TRUE, "ElevEncCnts"=0, "Action2"=enum."Wrist", "Action2Trigger"=0, "WristPositions"=enum."AllDown", "SlowRng"=2000.0, "TimeOut"=10.0, "GyroSens"=0.06, "DriveHeading"=350.0}, {"Action"=enum."Pause", "DriveEncCnts"=0, "Accel?"=FALSE, "Decel?"=FALSE, "ElevEncCnts"=0, "Action2"=enum."GripperToggle", "Action2Trigger"=0, "WristPositions"=enum."AllDown", "SlowRng"=0.0, "TimeOut"=0.5, "GyroSens"=0.0, "DriveHeading"=0.0}, {"Action"=enum."StraightBack", "DriveEncCnts"=-2000, "Accel?"=TRUE, "Decel?"=FALSE, "ElevEncCnts"=0, "Action2"=enum."", "Action2Trigger"=0, "WristPositions"=enum."AllDown", "SlowRng"=0.0, "TimeOut"=5.0, "GyroSens"=0.0, "DriveHeading"=0.0}, {"Action"=enum."StraightBack", "DriveEncCnts"=-1500, "Accel?"=FALSE, "Decel?"=TRUE, "ElevEncCnts"=0, "Action2"=enum."GripperToggle", "Action2Trigger"=0, "WristPositions"=enum."AllDown", "SlowRng"=-1200.0, "TimeOut"=5.0, "GyroSens"=0.002, "DriveHeading"=350.0}, {"Action"=enum."Pause", "DriveEncCnts"=0, "Accel?"=FALSE, "Decel?"=FALSE, "ElevEncCnts"=0, "Action2"=enum."", "Action2Trigger"=0, "WristPositions"=enum."AllDown", "SlowRng"=0.0, "TimeOut"=0.0, "GyroSens"=0.0, "DriveHeading"=0.0}, {"Action"=enum."GeneralTurn", "DriveEncCnts"=0, "Accel?"=FALSE, "Decel?"=FALSE, "ElevEncCnts"=0, "Action2"=enum."ElevDown", "Action2Trigger"=0, "WristPositions"=enum."AllDown", "SlowRng"=60.0, "TimeOut"=2.0, "GyroSens"=0.0, "DriveHeading"=190.0}, {"Action"=enum."StraightForward", "DriveEncCnts"=9000, "Accel?"=TRUE, "Decel?"=FALSE, "ElevEncCnts"=0, "Action2"=enum."ElevDown", "Action2Trigger"=0, "WristPositions"=enum."AllDown", "SlowRng"=7000.0, "TimeOut"=2.0, "GyroSens"=0.002, "DriveHeading"=190.0}, {"Action"=enum."StraightForward", "DriveEncCnts"=3000, "Accel?"=FALSE, "Decel?"=TRUE, "ElevEncCnts"=0, "Action2"=enum."Intake", "Action2Trigger"=0, "WristPositions"=enum."AllDown", "SlowRng"=1000.0, "TimeOut"=2.0, "GyroSens"=0.0, "DriveHeading"=190.0}, {"Action"=enum."Pause", "DriveEncCnts"=0, "Accel?"=FALSE, "Decel?"=FALSE, "ElevEncCnts"=0, "Action2"=enum."CubeCollect", "Action2Trigger"=0, "WristPositions"=enum."AllDown", "SlowRng"=0.0, "TimeOut"=0.5, "GyroSens"=0.0, "DriveHeading"=0.0}, {"Action"=enum."GeneralTurn", "DriveEncCnts"=0, "Accel?"=FALSE, "Decel?"=FALSE, "ElevEncCnts"=47000, "Action2"=enum."ElevUp", "Action2Trigger"=0, "WristPositions"=enum."AllDown", "SlowRng"=60.0, "TimeOut"=2.0, "GyroSens"=0.0, "DriveHeading"=350.0}, {"Action"=enum."StraightForward", "DriveEncCnts"=10000, "Accel?"=FALSE, "Decel?"=TRUE, "ElevEncCnts"=47000, "Action2"=enum."ElevUp", "Action2Trigger"=0, "WristPositions"=enum."AllDown", "SlowRng"=5000.0, "TimeOut"=1.5, "GyroSens"=0.002, "DriveHeading"=350.0}, {"Action"=enum."Pause", "DriveEncCnts"=0, "Accel?"=FALSE, "Decel?"=FALSE, "ElevEncCnts"=0, "Action2"=enum."ShifterToggle", "Action2Trigger"=0, "WristPositions"=enum."AllDown", "SlowRng"=0.0, "TimeOut"=0.0, "GyroSens"=0.0, "DriveHeading"=0.0}, {"Action"=enum."Stop", "DriveEncCnts"=0, "Accel?"=FALSE, "Decel?"=FALSE, "ElevEncCnts"=0, "Action2"=enum."GripperToggle", "Action2Trigger"=0, "WristPositions"=enum."AllDown", "SlowRng"=0.0, "TimeOut"=0.0, "GyroSens"=0.0, "DriveHeading"=0.0}, {"Action"=enum."Stop", "DriveEncCnts"=0, "Accel?"=FALSE, "Decel?"=FALSE, "ElevEncCnts"=0, "Action2"=enum."", "Action2Trigger"=0, "WristPositions"=enum."AllDown", "SlowRng"=0.0, "TimeOut"=0.0, "GyroSens"=0.0, "DriveHeading"=0.0}] T5 [{"Action"=enum."Initialize", "DriveEncCnts"=0, "Accel?"=FALSE, "Decel?"=FALSE, "ElevEncCnts"=0, "Action2"=enum."", "Action2Trigger"=0, "WristPositions"=enum."AllDown", "SlowRng"=0.0, "TimeOut"=0.0, "GyroSens"=0.0, "DriveHeading"=0.0}, {"Action"=enum."StraightForward", "DriveEncCnts"=93000, "Accel?"=TRUE, "Decel?"=TRUE, "ElevEncCnts"=0, "Action2"=enum."", "Action2Trigger"=0, "WristPositions"=enum."AllDown", "SlowRng"=50000.0, "TimeOut"=10.0, "GyroSens"=0.00065, "DriveHeading"=0.0}, {"Action"=enum."ForwardPivot", "DriveEncCnts"=0, "Accel?"=FALSE, "Decel?"=FALSE, "ElevEncCnts"=0, "Action2"=enum."", "Action2Trigger"=0, "WristPositions"=enum."AllDown", "SlowRng"=72.5, "TimeOut"=2.0, "GyroSens"=0.0, "DriveHeading"=270.0}, {"Action"=enum."StraightForward", "DriveEncCnts"=79000, "Accel?"=TRUE, "Decel?"=TRUE, "ElevEncCnts"=55000, "Action2"=enum."ElevUp", "Action2Trigger"=8000, "WristPositions"=enum."AllDown", "SlowRng"=25000.0, "TimeOut"=10.0, "GyroSens"=0.002, "DriveHeading"=270.0}, {"Action"=enum."ForwardPivot", "DriveEncCnts"=0, "Accel?"=FALSE, "Decel?"=FALSE, "ElevEncCnts"=0, "Action2"=enum."ShifterToggle", "Action2Trigger"=0, "WristPositions"=enum."AllDown", "SlowRng"=73.0, "TimeOut"=2.0, "GyroSens"=0.0, "DriveHeading"=10.0}, {"Action"=enum."StraightForward", "DriveEncCnts"=6000, "Accel?"=TRUE, "Decel?"=TRUE, "ElevEncCnts"=0, "Action2"=enum."Wrist", "Action2Trigger"=0, "WristPositions"=enum."AllDown", "SlowRng"=2000.0, "TimeOut"=10.0, "GyroSens"=0.06, "DriveHeading"=10.0}, {"Action"=enum."Pause", "DriveEncCnts"=0, "Accel?"=FALSE, "Decel?"=FALSE, "ElevEncCnts"=0, "Action2"=enum."GripperToggle", "Action2Trigger"=0, "WristPositions"=enum."AllDown", "SlowRng"=0.0, "TimeOut"=0.0, "GyroSens"=0.0, "DriveHeading"=0.0}, {"Action"=enum."StraightBack", "DriveEncCnts"=-2000, "Accel?"=TRUE, "Decel?"=FALSE, "ElevEncCnts"=0, "Action2"=enum."", "Action2Trigger"=0, "WristPositions"=enum."AllDown", "SlowRng"=0.0, "TimeOut"=5.0, "GyroSens"=0.0, "DriveHeading"=0.0}, {"Action"=enum."StraightBack", "DriveEncCnts"=-1500, "Accel?"=FALSE, "Decel?"=TRUE, "ElevEncCnts"=0, "Action2"=enum."GripperToggle", "Action2Trigger"=0, "WristPositions"=enum."AllDown", "SlowRng"=-1200.0, "TimeOut"=5.0, "GyroSens"=0.002, "DriveHeading"=10.0}, {"Action"=enum."Pause", "DriveEncCnts"=0, "Accel?"=FALSE, "Decel?"=FALSE, "ElevEncCnts"=0, "Action2"=enum."", "Action2Trigger"=0, "WristPositions"=enum."AllDown", "SlowRng"=0.0, "TimeOut"=0.0, "GyroSens"=0.0, "DriveHeading"=0.0}, {"Action"=enum."GeneralTurn", "DriveEncCnts"=0, "Accel?"=FALSE, "Decel?"=FALSE, "ElevEncCnts"=0, "Action2"=enum."ElevDown", "Action2Trigger"=0, "WristPositions"=enum."AllDown", "SlowRng"=60.0, "TimeOut"=2.0, "GyroSens"=0.0, "DriveHeading"=165.0}, {"Action"=enum."StraightForward", "DriveEncCnts"=9000, "Accel?"=TRUE, "Decel?"=FALSE, "ElevEncCnts"=0, "Action2"=enum."ElevDown", "Action2Trigger"=0, "WristPositions"=enum."AllDown", "SlowRng"=7000.0, "TimeOut"=2.0, "GyroSens"=0.002, "DriveHeading"=165.0}, {"Action"=enum."StraightForward", "DriveEncCnts"=3000, "Accel?"=FALSE, "Decel?"=TRUE, "ElevEncCnts"=0, "Action2"=enum."Intake", "Action2Trigger"=0, "WristPositions"=enum."AllDown", "SlowRng"=1000.0, "TimeOut"=2.0, "GyroSens"=0.0, "DriveHeading"=165.0}, {"Action"=enum."Pause", "DriveEncCnts"=0, "Accel?"=FALSE, "Decel?"=FALSE, "ElevEncCnts"=0, "Action2"=enum."CubeCollect", "Action2Trigger"=0, "WristPositions"=enum."AllDown", "SlowRng"=0.0, "TimeOut"=0.5, "GyroSens"=0.0, "DriveHeading"=0.0}, {"Action"=enum."GeneralTurn", "DriveEncCnts"=0, "Accel?"=FALSE, "Decel?"=FALSE, "ElevEncCnts"=47000, "Action2"=enum."ElevUp", "Action2Trigger"=0, "WristPositions"=enum."AllDown", "SlowRng"=60.0, "TimeOut"=2.0, "GyroSens"=0.0, "DriveHeading"=0.0}, {"Action"=enum."StraightForward", "DriveEncCnts"=10000, "Accel?"=FALSE, "Decel?"=TRUE, "ElevEncCnts"=47000, "Action2"=enum."ElevUp", "Action2Trigger"=0, "WristPositions"=enum."AllDown", "SlowRng"=5000.0, "TimeOut"=1.5, "GyroSens"=0.002, "DriveHeading"=0.0}, {"Action"=enum."Pause", "DriveEncCnts"=0, "Accel?"=FALSE, "Decel?"=FALSE, "ElevEncCnts"=0, "Action2"=enum."ShifterToggle", "Action2Trigger"=0, "WristPositions"=enum."AllDown", "SlowRng"=0.0, "TimeOut"=0.0, "GyroSens"=0.0, "DriveHeading"=0.0}, {"Action"=enum."Stop", "DriveEncCnts"=0, "Accel?"=FALSE, "Decel?"=FALSE, "ElevEncCnts"=0, "Action2"=enum."GripperToggle", "Action2Trigger"=0, "WristPositions"=enum."AllDown", "SlowRng"=0.0, "TimeOut"=0.0, "GyroSens"=0.0, "DriveHeading"=0.0}, {"Action"=enum."Stop", "DriveEncCnts"=0, "Accel?"=FALSE, "Decel?"=FALSE, "ElevEncCnts"=0, "Action2"=enum."", "Action2Trigger"=0, "WristPositions"=enum."AllDown", "SlowRng"=0.0, "TimeOut"=0.0, "GyroSens"=0.0, "DriveHeading"=0.0}] T5 [{"Action"=enum."Initialize", "DriveEncCnts"=0, "Accel?"=FALSE, "Decel?"=FALSE, "ElevEncCnts"=0, "Action2"=enum."", "Action2Trigger"=0, "WristPositions"=enum."AllDown", "SlowRng"=0.0, "TimeOut"=0.0, "GyroSens"=0.0, "DriveHeading"=0.0}, {"Action"=enum."StraightForward", "DriveEncCnts"=93000, "Accel?"=TRUE, "Decel?"=TRUE, "ElevEncCnts"=0, "Action2"=enum."", "Action2Trigger"=0, "WristPositions"=enum."AllDown", "SlowRng"=50000.0, "TimeOut"=10.0, "GyroSens"=0.00065, "DriveHeading"=0.0}, {"Action"=enum."ForwardPivot", "DriveEncCnts"=0, "Accel?"=FALSE, "Decel?"=FALSE, "ElevEncCnts"=0, "Action2"=enum."", "Action2Trigger"=0, "WristPositions"=enum."AllDown", "SlowRng"=70.0, "TimeOut"=2.0, "GyroSens"=0.0, "DriveHeading"=90.0}, {"Action"=enum."StraightForward", "DriveEncCnts"=78000, "Accel?"=TRUE, "Decel?"=TRUE, "ElevEncCnts"=55000, "Action2"=enum."ElevUp", "Action2Trigger"=8000, "WristPositions"=enum."AllDown", "SlowRng"=25000.0, "TimeOut"=10.0, "GyroSens"=0.02, "DriveHeading"=90.0}, {"Action"=enum."ForwardPivot", "DriveEncCnts"=0, "Accel?"=FALSE, "Decel?"=FALSE, "ElevEncCnts"=0, "Action2"=enum."ShifterToggle", "Action2Trigger"=0, "WristPositions"=enum."AllDown", "SlowRng"=70.0, "TimeOut"=2.0, "GyroSens"=0.0, "DriveHeading"=350.0}, {"Action"=enum."StraightForward", "DriveEncCnts"=6000, "Accel?"=TRUE, "Decel?"=TRUE, "ElevEncCnts"=0, "Action2"=enum."Wrist", "Action2Trigger"=0, "WristPositions"=enum."AllDown", "SlowRng"=2000.0, "TimeOut"=10.0, "GyroSens"=0.06, "DriveHeading"=350.0}, {"Action"=enum."Pause", "DriveEncCnts"=0, "Accel?"=FALSE, "Decel?"=FALSE, "ElevEncCnts"=0, "Action2"=enum."GripperToggle", "Action2Trigger"=0, "WristPositions"=enum."AllDown", "SlowRng"=0.0, "TimeOut"=0.5, "GyroSens"=0.0, "DriveHeading"=0.0}, {"Action"=enum."StraightBack", "DriveEncCnts"=-2000, "Accel?"=TRUE, "Decel?"=FALSE, "ElevEncCnts"=0, "Action2"=enum."", "Action2Trigger"=0, "WristPositions"=enum."AllDown", "SlowRng"=0.0, "TimeOut"=5.0, "GyroSens"=0.0, "DriveHeading"=0.0}, {"Action"=enum."StraightBack", "DriveEncCnts"=-1500, "Accel?"=FALSE, "Decel?"=TRUE, "ElevEncCnts"=0, "Action2"=enum."GripperToggle", "Action2Trigger"=0, "WristPositions"=enum."AllDown", "SlowRng"=-1200.0, "TimeOut"=5.0, "GyroSens"=0.002, "DriveHeading"=350.0}, {"Action"=enum."Pause", "DriveEncCnts"=0, "Accel?"=FALSE, "Decel?"=FALSE, "ElevEncCnts"=0, "Action2"=enum."", "Action2Trigger"=0, "WristPositions"=enum."AllDown", "SlowRng"=0.0, "TimeOut"=0.0, "GyroSens"=0.0, "DriveHeading"=0.0}, {"Action"=enum."GeneralTurn", "DriveEncCnts"=0, "Accel?"=FALSE, "Decel?"=FALSE, "ElevEncCnts"=0, "Action2"=enum."ElevDown", "Action2Trigger"=0, "WristPositions"=enum."AllDown", "SlowRng"=60.0, "TimeOut"=2.0, "GyroSens"=0.0, "DriveHeading"=190.0}, {"Action"=enum."StraightForward", "DriveEncCnts"=9000, "Accel?"=TRUE, "Decel?"=FALSE, "ElevEncCnts"=0, "Action2"=enum."ElevDown", "Action2Trigger"=0, "WristPositions"=enum."AllDown", "SlowRng"=7000.0, "TimeOut"=2.0, "GyroSens"=0.002, "DriveHeading"=190.0}, {"Action"=enum."StraightForward", "DriveEncCnts"=3000, "Accel?"=FALSE, "Decel?"=TRUE, "ElevEncCnts"=0, "Action2"=enum."Intake", "Action2Trigger"=0, "WristPositions"=enum."AllDown", "SlowRng"=1000.0, "TimeOut"=2.0, "GyroSens"=0.0, "DriveHeading"=190.0}, {"Action"=enum."Pause", "DriveEncCnts"=0, "Accel?"=FALSE, "Decel?"=FALSE, "ElevEncCnts"=0, "Action2"=enum."CubeCollect", "Action2Trigger"=0, "WristPositions"=enum."AllDown", "SlowRng"=0.0, "TimeOut"=0.5, "GyroSens"=0.0, "DriveHeading"=0.0}, {"Action"=enum."StraightBack", "DriveEncCnts"=-3000, "Accel?"=TRUE, "Decel?"=TRUE, "ElevEncCnts"=0, "Action2"=enum."Intake", "Action2Trigger"=0, "WristPositions"=enum."AllDown", "SlowRng"=-2000.0, "TimeOut"=5.0, "GyroSens"=0.002, "DriveHeading"=190.0}, {"Action"=enum."Pause", "DriveEncCnts"=0, "Accel?"=FALSE, "Decel?"=FALSE, "ElevEncCnts"=17000, "Action2"=enum."ElevUp", "Action2Trigger"=0, "WristPositions"=enum."AllDown", "SlowRng"=0.0, "TimeOut"=1.25, "GyroSens"=0.0, "DriveHeading"=0.0}, {"Action"=enum."StraightForward", "DriveEncCnts"=5000, "Accel?"=TRUE, "Decel?"=TRUE, "ElevEncCnts"=0, "Action2"=enum."ShifterToggle", "Action2Trigger"=0, "WristPositions"=enum."AllDown", "SlowRng"=2000.0, "TimeOut"=5.0, "GyroSens"=0.002, "DriveHeading"=190.0}, {"Action"=enum."Pause", "DriveEncCnts"=0, "Accel?"=FALSE, "Decel?"=FALSE, "ElevEncCnts"=0, "Action2"=enum."Release", "Action2Trigger"=0, "WristPositions"=enum."AllDown", "SlowRng"=0.0, "TimeOut"=1.5, "GyroSens"=0.0, "DriveHeading"=0.0}, {"Action"=enum."StraightBack", "DriveEncCnts"=-4500, "Accel?"=TRUE, "Decel?"=FALSE, "ElevEncCnts"=0, "Action2"=enum."ElevDown", "Action2Trigger"=0, "WristPositions"=enum."AllDown", "SlowRng"=-2000.0, "TimeOut"=3.0, "GyroSens"=0.002, "DriveHeading"=270.0}, {"Action"=enum."StraightBack", "DriveEncCnts"=-6000, "Accel?"=FALSE, "Decel?"=TRUE, "ElevEncCnts"=0, "Action2"=enum."", "Action2Trigger"=0, "WristPositions"=enum."AllDown", "SlowRng"=-1250.0, "TimeOut"=3.0, "GyroSens"=0.002, "DriveHeading"=270.0}, {"Action"=enum."Stop", "DriveEncCnts"=0, "Accel?"=TRUE, "Decel?"=TRUE, "ElevEncCnts"=0, "Action2"=enum."", "Action2Trigger"=0, "WristPositions"=enum."AllDown", "SlowRng"=0.0, "TimeOut"=0.0, "GyroSens"=0.0, "DriveHeading"=0.0}] T5 [{"Action"=enum."Initialize", "DriveEncCnts"=0, "Accel?"=FALSE, "Decel?"=FALSE, "ElevEncCnts"=0, "Action2"=enum."", "Action2Trigger"=0, "WristPositions"=enum."AllDown", "SlowRng"=0.0, "TimeOut"=0.0, "GyroSens"=0.0, "DriveHeading"=0.0}, {"Action"=enum."StraightForward", "DriveEncCnts"=93000, "Accel?"=TRUE, "Decel?"=TRUE, "ElevEncCnts"=0, "Action2"=enum."", "Action2Trigger"=0, "WristPositions"=enum."AllDown", "SlowRng"=50000.0, "TimeOut"=10.0, "GyroSens"=0.00065, "DriveHeading"=0.0}, {"Action"=enum."ForwardPivot", "DriveEncCnts"=0, "Accel?"=FALSE, "Decel?"=FALSE, "ElevEncCnts"=0, "Action2"=enum."", "Action2Trigger"=0, "WristPositions"=enum."AllDown", "SlowRng"=72.5, "TimeOut"=2.0, "GyroSens"=0.0, "DriveHeading"=270.0}, {"Action"=enum."StraightForward", "DriveEncCnts"=76000, "Accel?"=TRUE, "Decel?"=TRUE, "ElevEncCnts"=55000, "Action2"=enum."ElevUp", "Action2Trigger"=8000, "WristPositions"=enum."AllDown", "SlowRng"=25000.0, "TimeOut"=10.0, "GyroSens"=0.02, "DriveHeading"=270.0}, {"Action"=enum."ForwardPivot", "DriveEncCnts"=0, "Accel?"=FALSE, "Decel?"=FALSE, "ElevEncCnts"=0, "Action2"=enum."ShifterToggle", "Action2Trigger"=0, "WristPositions"=enum."AllDown", "SlowRng"=73.0, "TimeOut"=2.0, "GyroSens"=0.0, "DriveHeading"=10.0}, {"Action"=enum."StraightForward", "DriveEncCnts"=6000, "Accel?"=TRUE, "Decel?"=TRUE, "ElevEncCnts"=0, "Action2"=enum."Wrist", "Action2Trigger"=0, "WristPositions"=enum."AllDown", "SlowRng"=2000.0, "TimeOut"=10.0, "GyroSens"=0.06, "DriveHeading"=10.0}, {"Action"=enum."Pause", "DriveEncCnts"=0, "Accel?"=FALSE, "Decel?"=FALSE, "ElevEncCnts"=0, "Action2"=enum."GripperToggle", "Action2Trigger"=0, "WristPositions"=enum."AllDown", "SlowRng"=0.0, "TimeOut"=0.0, "GyroSens"=0.0, "DriveHeading"=0.0}, {"Action"=enum."StraightBack", "DriveEncCnts"=-2000, "Accel?"=TRUE, "Decel?"=FALSE, "ElevEncCnts"=0, "Action2"=enum."", "Action2Trigger"=0, "WristPositions"=enum."AllDown", "SlowRng"=0.0, "TimeOut"=5.0, "GyroSens"=0.0, "DriveHeading"=0.0}, {"Action"=enum."StraightBack", "DriveEncCnts"=-1500, "Accel?"=FALSE, "Decel?"=TRUE, "ElevEncCnts"=0, "Action2"=enum."GripperToggle", "Action2Trigger"=0, "WristPositions"=enum."AllDown", "SlowRng"=-1200.0, "TimeOut"=5.0, "GyroSens"=0.002, "DriveHeading"=10.0}, {"Action"=enum."Pause", "DriveEncCnts"=0, "Accel?"=FALSE, "Decel?"=FALSE, "ElevEncCnts"=0, "Action2"=enum."", "Action2Trigger"=0, "WristPositions"=enum."AllDown", "SlowRng"=0.0, "TimeOut"=0.0, "GyroSens"=0.0, "DriveHeading"=0.0}, {"Action"=enum."GeneralTurn", "DriveEncCnts"=0, "Accel?"=FALSE, "Decel?"=FALSE, "ElevEncCnts"=0, "Action2"=enum."ElevDown", "Action2Trigger"=0, "WristPositions"=enum."AllDown", "SlowRng"=60.0, "TimeOut"=2.0, "GyroSens"=0.0, "DriveHeading"=165.0}, {"Action"=enum."StraightForward", "DriveEncCnts"=9000, "Accel?"=TRUE, "Decel?"=FALSE, "ElevEncCnts"=0, "Action2"=enum."ElevDown", "Action2Trigger"=0, "WristPositions"=enum."AllDown", "SlowRng"=7000.0, "TimeOut"=2.0, "GyroSens"=0.002, "DriveHeading"=165.0}, {"Action"=enum."StraightForward", "DriveEncCnts"=3000, "Accel?"=FALSE, "Decel?"=TRUE, "ElevEncCnts"=0, "Action2"=enum."Intake", "Action2Trigger"=0, "WristPositions"=enum."AllDown", "SlowRng"=1000.0, "TimeOut"=2.0, "GyroSens"=0.0, "DriveHeading"=165.0}, {"Action"=enum."Pause", "DriveEncCnts"=0, "Accel?"=FALSE, "Decel?"=FALSE, "ElevEncCnts"=0, "Action2"=enum."CubeCollect", "Action2Trigger"=0, "WristPositions"=enum."AllDown", "SlowRng"=0.0, "TimeOut"=0.5, "GyroSens"=0.0, "DriveHeading"=0.0}, {"Action"=enum."StraightBack", "DriveEncCnts"=-3000, "Accel?"=TRUE, "Decel?"=TRUE, "ElevEncCnts"=0, "Action2"=enum."Intake", "Action2Trigger"=0, "WristPositions"=enum."AllDown", "SlowRng"=-2000.0, "TimeOut"=5.0, "GyroSens"=0.002, "DriveHeading"=165.0}, {"Action"=enum."Pause", "DriveEncCnts"=0, "Accel?"=FALSE, "Decel?"=FALSE, "ElevEncCnts"=17000, "Action2"=enum."ElevUp", "Action2Trigger"=0, "WristPositions"=enum."AllDown", "SlowRng"=0.0, "TimeOut"=1.25, "GyroSens"=0.0, "DriveHeading"=0.0}, {"Action"=enum."StraightForward", "DriveEncCnts"=5000, "Accel?"=TRUE, "Decel?"=TRUE, "ElevEncCnts"=0, "Action2"=enum."ShifterToggle", "Action2Trigger"=0, "WristPositions"=enum."AllDown", "SlowRng"=2000.0, "TimeOut"=5.0, "GyroSens"=0.002, "DriveHeading"=165.0}, {"Action"=enum."Pause", "DriveEncCnts"=0, "Accel?"=FALSE, "Decel?"=FALSE, "ElevEncCnts"=0, "Action2"=enum."Release", "Action2Trigger"=0, "WristPositions"=enum."AllDown", "SlowRng"=0.0, "TimeOut"=1.5, "GyroSens"=0.0, "DriveHeading"=0.0}, {"Action"=enum."StraightBack", "DriveEncCnts"=-4500, "Accel?"=TRUE, "Decel?"=FALSE, "ElevEncCnts"=0, "Action2"=enum."ElevDown", "Action2Trigger"=0, "WristPositions"=enum."AllDown", "SlowRng"=-2000.0, "TimeOut"=3.0, "GyroSens"=0.002, "DriveHeading"=90.0}, {"Action"=enum."StraightBack", "DriveEncCnts"=-6000, "Accel?"=FALSE, "Decel?"=TRUE, "ElevEncCnts"=0, "Action2"=enum."", "Action2Trigger"=0, "WristPositions"=enum."AllDown", "SlowRng"=-1250.0, "TimeOut"=3.0, "GyroSens"=0.002, "DriveHeading"=90.0}, {"Action"=enum."Stop", "DriveEncCnts"=0, "Accel?"=FALSE, "Decel?"=FALSE, "ElevEncCnts"=0, "Action2"=enum."", "Action2Trigger"=0, "WristPositions"=enum."AllDown", "SlowRng"=0.0, "TimeOut"=0.0, "GyroSens"=0.0, "DriveHeading"=0.0}] T5 [{"Action"=enum."Initialize", "DriveEncCnts"=0, "Accel?"=FALSE, "Decel?"=FALSE, "ElevEncCnts"=0, "Action2"=enum."", "Action2Trigger"=0, "WristPositions"=enum."AllDown", "SlowRng"=0.0, "TimeOut"=0.0, "GyroSens"=0.0, "DriveHeading"=0.0}, {"Action"=enum."StraightForward", "DriveEncCnts"=105000, "Accel?"=TRUE, "Decel?"=TRUE, "ElevEncCnts"=55000, "Action2"=enum."ElevUp", "Action2Trigger"=25000, "WristPositions"=enum."AllDown", "SlowRng"=35000.0, "TimeOut"=10.0, "GyroSens"=0.00065, "DriveHeading"=0.0}, {"Action"=enum."ForwardPivot", "DriveEncCnts"=0, "Accel?"=FALSE, "Decel?"=FALSE, "ElevEncCnts"=0, "Action2"=enum."ShifterToggle", "Action2Trigger"=0, "WristPositions"=enum."AllDown", "SlowRng"=57.0, "TimeOut"=1.5, "GyroSens"=0.0, "DriveHeading"=45.0}, {"Action"=enum."StraightForward", "DriveEncCnts"=8000, "Accel?"=FALSE, "Decel?"=TRUE, "ElevEncCnts"=0, "Action2"=enum."", "Action2Trigger"=0, "WristPositions"=enum."AllDown", "SlowRng"=4000.0, "TimeOut"=10.0, "GyroSens"=0.05, "DriveHeading"=45.0}, {"Action"=enum."Pause", "DriveEncCnts"=0, "Accel?"=FALSE, "Decel?"=FALSE, "ElevEncCnts"=0, "Action2"=enum."Wrist", "Action2Trigger"=0, "WristPositions"=enum."AllDown", "SlowRng"=0.0, "TimeOut"=0.25, "GyroSens"=0.0, "DriveHeading"=0.0}, {"Action"=enum."Pause", "DriveEncCnts"=0, "Accel?"=FALSE, "Decel?"=FALSE, "ElevEncCnts"=0, "Action2"=enum."Release", "Action2Trigger"=0, "WristPositions"=enum."AllDown", "SlowRng"=0.0, "TimeOut"=0.5, "GyroSens"=0.0, "DriveHeading"=0.0}, {"Action"=enum."StraightBack", "DriveEncCnts"=-8000, "Accel?"=TRUE, "Decel?"=TRUE, "ElevEncCnts"=0, "Action2"=enum."", "Action2Trigger"=0, "WristPositions"=enum."AllDown", "SlowRng"=-4000.0, "TimeOut"=5.0, "GyroSens"=0.05, "DriveHeading"=45.0}, {"Action"=enum."BackPivot", "DriveEncCnts"=0, "Accel?"=FALSE, "Decel?"=FALSE, "ElevEncCnts"=0, "Action2"=enum."ElevDown", "Action2Trigger"=0, "WristPositions"=enum."AllDown", "SlowRng"=28.0, "TimeOut"=1.5, "GyroSens"=0.0, "DriveHeading"=90.0}, {"Action"=enum."ForwardPivot", "DriveEncCnts"=0, "Accel?"=FALSE, "Decel?"=FALSE, "ElevEncCnts"=0, "Action2"=enum."ElevDown", "Action2Trigger"=0, "WristPositions"=enum."AllDown", "SlowRng"=36.0, "TimeOut"=1.75, "GyroSens"=0.0, "DriveHeading"=135.0}, {"Action"=enum."StraightForward", "DriveEncCnts"=9500, "Accel?"=FALSE, "Decel?"=FALSE, "ElevEncCnts"=0, "Action2"=enum."ElevDown", "Action2Trigger"=0, "WristPositions"=enum."AllDown", "SlowRng"=0.0, "TimeOut"=10.0, "GyroSens"=0.006, "DriveHeading"=135.0}, {"Action"=enum."StraightForward", "DriveEncCnts"=5000, "Accel?"=FALSE, "Decel?"=TRUE, "ElevEncCnts"=0, "Action2"=enum."Intake", "Action2Trigger"=0, "WristPositions"=enum."AllDown", "SlowRng"=6000.0, "TimeOut"=10.0, "GyroSens"=0.00065, "DriveHeading"=135.0}, {"Action"=enum."Pause", "DriveEncCnts"=0, "Accel?"=FALSE, "Decel?"=FALSE, "ElevEncCnts"=0, "Action2"=enum."CubeCollect", "Action2Trigger"=0, "WristPositions"=enum."AllDown", "SlowRng"=0.0, "TimeOut"=0.5, "GyroSens"=0.0, "DriveHeading"=0.0}, {"Action"=enum."StraightBack", "DriveEncCnts"=-14500, "Accel?"=TRUE, "Decel?"=TRUE, "ElevEncCnts"=0, "Action2"=enum."Intake", "Action2Trigger"=0, "WristPositions"=enum."AllDown", "SlowRng"=-12000.0, "TimeOut"=10.0, "GyroSens"=0.00065, "DriveHeading"=135.0}, {"Action"=enum."BackPivot", "DriveEncCnts"=0, "Accel?"=FALSE, "Decel?"=FALSE, "ElevEncCnts"=47000, "Action2"=enum."ElevUp", "Action2Trigger"=0, "WristPositions"=enum."AllDown", "SlowRng"=32.0, "TimeOut"=1.25, "GyroSens"=0.0, "DriveHeading"=90.0}, {"Action"=enum."ForwardPivot", "DriveEncCnts"=0, "Accel?"=FALSE, "Decel?"=FALSE, "ElevEncCnts"=47000, "Action2"=enum."ElevUp", "Action2Trigger"=0, "WristPositions"=enum."AllDown", "SlowRng"=45.0, "TimeOut"=1.25, "GyroSens"=0.0, "DriveHeading"=35.0}, {"Action"=enum."StraightForward", "DriveEncCnts"=17000, "Accel?"=TRUE, "Decel?"=TRUE, "ElevEncCnts"=0, "Action2"=enum."ShifterToggle", "Action2Trigger"=0, "WristPositions"=enum."AllDown", "SlowRng"=6000.0, "TimeOut"=1.5, "GyroSens"=0.05, "DriveHeading"=35.0}, {"Action"=enum."Pause", "DriveEncCnts"=0, "Accel?"=FALSE, "Decel?"=FALSE, "ElevEncCnts"=0, "Action2"=enum."GripperToggle", "Action2Trigger"=0, "WristPositions"=enum."AllDown", "SlowRng"=0.0, "TimeOut"=0.25, "GyroSens"=0.0, "DriveHeading"=0.0}, {"Action"=enum."StraightBack", "DriveEncCnts"=-10000, "Accel?"=TRUE, "Decel?"=TRUE, "ElevEncCnts"=0, "Action2"=enum."", "Action2Trigger"=0, "WristPositions"=enum."AllDown", "SlowRng"=-6000.0, "TimeOut"=1.5, "GyroSens"=0.0, "DriveHeading"=37.0}, {"Action"=enum."Stop", "DriveEncCnts"=0, "Accel?"=FALSE, "Decel?"=FALSE, "ElevEncCnts"=0, "Action2"=enum."ElevDown", "Action2Trigger"=0, "WristPositions"=enum."AllDown", "SlowRng"=0.0, "TimeOut"=0.0, "GyroSens"=0.0, "DriveHeading"=0.0}] T5 [{"Action"=enum."Initialize", "DriveEncCnts"=0, "Accel?"=FALSE, "Decel?"=FALSE, "ElevEncCnts"=0, "Action2"=enum."", "Action2Trigger"=0, "WristPositions"=enum."AllDown", "SlowRng"=0.0, "TimeOut"=0.0, "GyroSens"=0.0, "DriveHeading"=0.0}, {"Action"=enum."StraightForward", "DriveEncCnts"=101000, "Accel?"=TRUE, "Decel?"=TRUE, "ElevEncCnts"=55000, "Action2"=enum."ElevUp", "Action2Trigger"=25000, "WristPositions"=enum."AllDown", "SlowRng"=35000.0, "TimeOut"=10.0, "GyroSens"=0.00065, "DriveHeading"=0.0}, {"Action"=enum."ForwardPivot", "DriveEncCnts"=0, "Accel?"=FALSE, "Decel?"=FALSE, "ElevEncCnts"=0, "Action2"=enum."ShifterToggle", "Action2Trigger"=0, "WristPositions"=enum."AllDown", "SlowRng"=57.0, "TimeOut"=1.5, "GyroSens"=0.0, "DriveHeading"=315.0}, {"Action"=enum."StraightForward", "DriveEncCnts"=7500, "Accel?"=FALSE, "Decel?"=TRUE, "ElevEncCnts"=0, "Action2"=enum."", "Action2Trigger"=0, "WristPositions"=enum."AllDown", "SlowRng"=4000.0, "TimeOut"=10.0, "GyroSens"=0.05, "DriveHeading"=315.0}, {"Action"=enum."Pause", "DriveEncCnts"=0, "Accel?"=FALSE, "Decel?"=FALSE, "ElevEncCnts"=0, "Action2"=enum."Wrist", "Action2Trigger"=0, "WristPositions"=enum."AllDown", "SlowRng"=0.0, "TimeOut"=0.25, "GyroSens"=0.0, "DriveHeading"=0.0}, {"Action"=enum."Pause", "DriveEncCnts"=0, "Accel?"=FALSE, "Decel?"=FALSE, "ElevEncCnts"=0, "Action2"=enum."Release", "Action2Trigger"=0, "WristPositions"=enum."AllDown", "SlowRng"=0.0, "TimeOut"=0.5, "GyroSens"=0.0, "DriveHeading"=0.0}, {"Action"=enum."StraightBack", "DriveEncCnts"=-9000, "Accel?"=TRUE, "Decel?"=TRUE, "ElevEncCnts"=0, "Action2"=enum."", "Action2Trigger"=0, "WristPositions"=enum."AllDown", "SlowRng"=-6000.0, "TimeOut"=5.0, "GyroSens"=0.05, "DriveHeading"=315.0}, {"Action"=enum."BackPivot", "DriveEncCnts"=0, "Accel?"=FALSE, "Decel?"=FALSE, "ElevEncCnts"=0, "Action2"=enum."ElevDown", "Action2Trigger"=0, "WristPositions"=enum."AllDown", "SlowRng"=28.0, "TimeOut"=1.5, "GyroSens"=0.0, "DriveHeading"=270.0}, {"Action"=enum."ForwardPivot", "DriveEncCnts"=0, "Accel?"=FALSE, "Decel?"=FALSE, "ElevEncCnts"=0, "Action2"=enum."ElevDown", "Action2Trigger"=0, "WristPositions"=enum."AllDown", "SlowRng"=36.0, "TimeOut"=1.75, "GyroSens"=0.0, "DriveHeading"=225.0}, {"Action"=enum."StraightForward", "DriveEncCnts"=9500, "Accel?"=FALSE, "Decel?"=FALSE, "ElevEncCnts"=0, "Action2"=enum."ElevDown", "Action2Trigger"=0, "WristPositions"=enum."AllDown", "SlowRng"=0.0, "TimeOut"=10.0, "GyroSens"=0.006, "DriveHeading"=225.0}, {"Action"=enum."StraightForward", "DriveEncCnts"=5000, "Accel?"=FALSE, "Decel?"=TRUE, "ElevEncCnts"=0, "Action2"=enum."Intake", "Action2Trigger"=0, "WristPositions"=enum."AllDown", "SlowRng"=6000.0, "TimeOut"=10.0, "GyroSens"=0.00065, "DriveHeading"=225.0}, {"Action"=enum."Pause", "DriveEncCnts"=0, "Accel?"=FALSE, "Decel?"=FALSE, "ElevEncCnts"=0, "Action2"=enum."CubeCollect", "Action2Trigger"=0, "WristPositions"=enum."AllDown", "SlowRng"=0.0, "TimeOut"=0.5, "GyroSens"=0.0, "DriveHeading"=0.0}, {"Action"=enum."StraightBack", "DriveEncCnts"=-14500, "Accel?"=TRUE, "Decel?"=TRUE, "ElevEncCnts"=0, "Action2"=enum."Intake", "Action2Trigger"=0, "WristPositions"=enum."AllDown", "SlowRng"=-12000.0, "TimeOut"=10.0, "GyroSens"=0.00065, "DriveHeading"=225.0}, {"Action"=enum."BackPivot", "DriveEncCnts"=0, "Accel?"=FALSE, "Decel?"=FALSE, "ElevEncCnts"=49000, "Action2"=enum."ElevUp", "Action2Trigger"=0, "WristPositions"=enum."AllDown", "SlowRng"=32.0, "TimeOut"=1.25, "GyroSens"=0.0, "DriveHeading"=270.0}, {"Action"=enum."ForwardPivot", "DriveEncCnts"=0, "Accel?"=FALSE, "Decel?"=FALSE, "ElevEncCnts"=49000, "Action2"=enum."ElevUp", "Action2Trigger"=0, "WristPositions"=enum."AllDown", "SlowRng"=45.0, "TimeOut"=1.25, "GyroSens"=0.0, "DriveHeading"=310.0}, {"Action"=enum."StraightForward", "DriveEncCnts"=17000, "Accel?"=FALSE, "Decel?"=TRUE, "ElevEncCnts"=0, "Action2"=enum."ShifterToggle", "Action2Trigger"=0, "WristPositions"=enum."AllDown", "SlowRng"=6000.0, "TimeOut"=1.5, "GyroSens"=0.05, "DriveHeading"=310.0}, {"Action"=enum."Pause", "DriveEncCnts"=0, "Accel?"=FALSE, "Decel?"=FALSE, "ElevEncCnts"=0, "Action2"=enum."GripperToggle", "Action2Trigger"=0, "WristPositions"=enum."AllDown", "SlowRng"=0.0, "TimeOut"=0.25, "GyroSens"=0.0, "DriveHeading"=0.0}, {"Action"=enum."StraightBack", "DriveEncCnts"=-10000, "Accel?"=TRUE, "Decel?"=TRUE, "ElevEncCnts"=0, "Action2"=enum."", "Action2Trigger"=0, "WristPositions"=enum."AllDown", "SlowRng"=-6000.0, "TimeOut"=1.5, "GyroSens"=0.0, "DriveHeading"=315.0}, {"Action"=enum."Stop", "DriveEncCnts"=0, "Accel?"=FALSE, "Decel?"=FALSE, "ElevEncCnts"=0, "Action2"=enum."ElevDown", "Action2Trigger"=0, "WristPositions"=enum."AllDown", "SlowRng"=0.0, "TimeOut"=0.0, "GyroSens"=0.0, "DriveHeading"=0.0}] T5 [{"Action"=enum."Initialize", "DriveEncCnts"=0, "Accel?"=FALSE, "Decel?"=FALSE, "ElevEncCnts"=0, "Action2"=enum."", "Action2Trigger"=0, "WristPositions"=enum."AllDown", "SlowRng"=0.0, "TimeOut"=0.0, "GyroSens"=0.0, "DriveHeading"=0.0}, {"Action"=enum."StraightForward", "DriveEncCnts"=105000, "Accel?"=TRUE, "Decel?"=TRUE, "ElevEncCnts"=55000, "Action2"=enum."ElevUp", "Action2Trigger"=25000, "WristPositions"=enum."AllDown", "SlowRng"=35000.0, "TimeOut"=10.0, "GyroSens"=0.00065, "DriveHeading"=0.0}, {"Action"=enum."ForwardPivot", "DriveEncCnts"=0, "Accel?"=FALSE, "Decel?"=FALSE, "ElevEncCnts"=0, "Action2"=enum."ShifterToggle", "Action2Trigger"=0, "WristPositions"=enum."AllDown", "SlowRng"=57.0, "TimeOut"=1.5, "GyroSens"=0.0, "DriveHeading"=45.0}, {"Action"=enum."StraightForward", "DriveEncCnts"=8000, "Accel?"=FALSE, "Decel?"=TRUE, "ElevEncCnts"=0, "Action2"=enum."", "Action2Trigger"=0, "WristPositions"=enum."AllDown", "SlowRng"=4000.0, "TimeOut"=10.0, "GyroSens"=0.05, "DriveHeading"=45.0}, {"Action"=enum."Pause", "DriveEncCnts"=0, "Accel?"=FALSE, "Decel?"=FALSE, "ElevEncCnts"=0, "Action2"=enum."Wrist", "Action2Trigger"=0, "WristPositions"=enum."AllDown", "SlowRng"=0.0, "TimeOut"=0.25, "GyroSens"=0.0, "DriveHeading"=0.0}, {"Action"=enum."Pause", "DriveEncCnts"=0, "Accel?"=FALSE, "Decel?"=FALSE, "ElevEncCnts"=0, "Action2"=enum."Release", "Action2Trigger"=0, "WristPositions"=enum."AllDown", "SlowRng"=0.0, "TimeOut"=0.5, "GyroSens"=0.0, "DriveHeading"=0.0}, {"Action"=enum."StraightBack", "DriveEncCnts"=-8000, "Accel?"=TRUE, "Decel?"=TRUE, "ElevEncCnts"=0, "Action2"=enum."", "Action2Trigger"=0, "WristPositions"=enum."AllDown", "SlowRng"=-4000.0, "TimeOut"=5.0, "GyroSens"=0.05, "DriveHeading"=45.0}, {"Action"=enum."BackPivot", "DriveEncCnts"=0, "Accel?"=FALSE, "Decel?"=FALSE, "ElevEncCnts"=0, "Action2"=enum."ElevDown", "Action2Trigger"=0, "WristPositions"=enum."AllDown", "SlowRng"=28.0, "TimeOut"=1.5, "GyroSens"=0.0, "DriveHeading"=90.0}, {"Action"=enum."ForwardPivot", "DriveEncCnts"=0, "Accel?"=FALSE, "Decel?"=FALSE, "ElevEncCnts"=0, "Action2"=enum."ElevDown", "Action2Trigger"=0, "WristPositions"=enum."AllDown", "SlowRng"=36.0, "TimeOut"=1.75, "GyroSens"=0.0, "DriveHeading"=145.0}, {"Action"=enum."StraightForward", "DriveEncCnts"=9500, "Accel?"=TRUE, "Decel?"=FALSE, "ElevEncCnts"=0, "Action2"=enum."ElevDown", "Action2Trigger"=0, "WristPositions"=enum."AllDown", "SlowRng"=0.0, "TimeOut"=10.0, "GyroSens"=0.006, "DriveHeading"=145.0}, {"Action"=enum."StraightForward", "DriveEncCnts"=7000, "Accel?"=FALSE, "Decel?"=TRUE, "ElevEncCnts"=0, "Action2"=enum."Intake", "Action2Trigger"=0, "WristPositions"=enum."AllDown", "SlowRng"=6000.0, "TimeOut"=10.0, "GyroSens"=0.00065, "DriveHeading"=145.0}, {"Action"=enum."Pause", "DriveEncCnts"=0, "Accel?"=FALSE, "Decel?"=FALSE, "ElevEncCnts"=0, "Action2"=enum."CubeCollect", "Action2Trigger"=0, "WristPositions"=enum."AllDown", "SlowRng"=0.0, "TimeOut"=0.5, "GyroSens"=0.0, "DriveHeading"=0.0}, {"Action"=enum."StraightBack", "DriveEncCnts"=-5000, "Accel?"=TRUE, "Decel?"=TRUE, "ElevEncCnts"=0, "Action2"=enum."Intake", "Action2Trigger"=0, "WristPositions"=enum."AllDown", "SlowRng"=-2000.0, "TimeOut"=10.0, "GyroSens"=0.00065, "DriveHeading"=145.0}, {"Action"=enum."Pause", "DriveEncCnts"=0, "Accel?"=FALSE, "Decel?"=FALSE, "ElevEncCnts"=17000, "Action2"=enum."ElevUp", "Action2Trigger"=0, "WristPositions"=enum."AllDown", "SlowRng"=0.0, "TimeOut"=1.0, "GyroSens"=0.0, "DriveHeading"=0.0}, {"Action"=enum."StraightForward", "DriveEncCnts"=7000, "Accel?"=TRUE, "Decel?"=TRUE, "ElevEncCnts"=0, "Action2"=enum."ShifterToggle", "Action2Trigger"=0, "WristPositions"=enum."AllDown", "SlowRng"=2000.0, "TimeOut"=1.5, "GyroSens"=0.00065, "DriveHeading"=145.0}, {"Action"=enum."Pause", "DriveEncCnts"=0, "Accel?"=FALSE, "Decel?"=FALSE, "ElevEncCnts"=0, "Action2"=enum."Release", "Action2Trigger"=0, "WristPositions"=enum."AllDown", "SlowRng"=0.0, "TimeOut"=1.5, "GyroSens"=0.0, "DriveHeading"=0.0}, {"Action"=enum."BackPivot", "DriveEncCnts"=0, "Accel?"=FALSE, "Decel?"=FALSE, "ElevEncCnts"=0, "Action2"=enum."GripperToggle", "Action2Trigger"=0, "WristPositions"=enum."AllDown", "SlowRng"=30.0, "TimeOut"=0.25, "GyroSens"=0.0, "DriveHeading"=112.5}, {"Action"=enum."Pause", "DriveEncCnts"=0, "Accel?"=FALSE, "Decel?"=FALSE, "ElevEncCnts"=0, "Action2"=enum."ElevDown", "Action2Trigger"=0, "WristPositions"=enum."AllDown", "SlowRng"=0.0, "TimeOut"=1.0, "GyroSens"=0.0, "DriveHeading"=0.0}, {"Action"=enum."StraightForward", "DriveEncCnts"=5000, "Accel?"=TRUE, "Decel?"=TRUE, "ElevEncCnts"=0, "Action2"=enum."Intake", "Action2Trigger"=0, "WristPositions"=enum."AllDown", "SlowRng"=2000.0, "TimeOut"=1.5, "GyroSens"=0.00065, "DriveHeading"=112.5}, {"Action"=enum."Pause", "DriveEncCnts"=0, "Accel?"=FALSE, "Decel?"=FALSE, "ElevEncCnts"=0, "Action2"=enum."CubeCollect", "Action2Trigger"=0, "WristPositions"=enum."AllDown", "SlowRng"=0.0, "TimeOut"=0.5, "GyroSens"=0.0, "DriveHeading"=0.0}, {"Action"=enum."StraightBack", "DriveEncCnts"=-10000, "Accel?"=TRUE, "Decel?"=TRUE, "ElevEncCnts"=0, "Action2"=enum."Intake", "Action2Trigger"=0, "WristPositions"=enum."AllDown", "SlowRng"=-7500.0, "TimeOut"=5.0, "GyroSens"=0.00065, "DriveHeading"=90.0}] T5 [{"Action"=enum."Initialize", "DriveEncCnts"=0, "Accel?"=FALSE, "Decel?"=FALSE, "ElevEncCnts"=0, "Action2"=enum."", "Action2Trigger"=0, "WristPositions"=enum."AllDown", "SlowRng"=0.0, "TimeOut"=0.0, "GyroSens"=0.0, "DriveHeading"=0.0}, {"Action"=enum."StraightForward", "DriveEncCnts"=101000, "Accel?"=TRUE, "Decel?"=TRUE, "ElevEncCnts"=55000, "Action2"=enum."ElevUp", "Action2Trigger"=25000, "WristPositions"=enum."AllDown", "SlowRng"=35000.0, "TimeOut"=10.0, "GyroSens"=0.00065, "DriveHeading"=0.0}, {"Action"=enum."ForwardPivot", "DriveEncCnts"=0, "Accel?"=FALSE, "Decel?"=FALSE, "ElevEncCnts"=0, "Action2"=enum."ShifterToggle", "Action2Trigger"=0, "WristPositions"=enum."AllDown", "SlowRng"=57.0, "TimeOut"=1.5, "GyroSens"=0.0, "DriveHeading"=315.0}, {"Action"=enum."StraightForward", "DriveEncCnts"=7500, "Accel?"=FALSE, "Decel?"=TRUE, "ElevEncCnts"=0, "Action2"=enum."", "Action2Trigger"=0, "WristPositions"=enum."AllDown", "SlowRng"=4000.0, "TimeOut"=10.0, "GyroSens"=0.05, "DriveHeading"=315.0}, {"Action"=enum."Pause", "DriveEncCnts"=0, "Accel?"=FALSE, "Decel?"=FALSE, "ElevEncCnts"=0, "Action2"=enum."Wrist", "Action2Trigger"=0, "WristPositions"=enum."AllDown", "SlowRng"=0.0, "TimeOut"=0.25, "GyroSens"=0.0, "DriveHeading"=0.0}, {"Action"=enum."Pause", "DriveEncCnts"=0, "Accel?"=FALSE, "Decel?"=FALSE, "ElevEncCnts"=0, "Action2"=enum."Release", "Action2Trigger"=0, "WristPositions"=enum."AllDown", "SlowRng"=0.0, "TimeOut"=0.5, "GyroSens"=0.0, "DriveHeading"=0.0}, {"Action"=enum."StraightBack", "DriveEncCnts"=-9000, "Accel?"=TRUE, "Decel?"=TRUE, "ElevEncCnts"=0, "Action2"=enum."", "Action2Trigger"=0, "WristPositions"=enum."AllDown", "SlowRng"=-6000.0, "TimeOut"=5.0, "GyroSens"=0.05, "DriveHeading"=315.0}, {"Action"=enum."BackPivot", "DriveEncCnts"=0, "Accel?"=FALSE, "Decel?"=FALSE, "ElevEncCnts"=0, "Action2"=enum."ElevDown", "Action2Trigger"=0, "WristPositions"=enum."AllDown", "SlowRng"=28.0, "TimeOut"=1.5, "GyroSens"=0.0, "DriveHeading"=270.0}, {"Action"=enum."ForwardPivot", "DriveEncCnts"=0, "Accel?"=FALSE, "Decel?"=FALSE, "ElevEncCnts"=0, "Action2"=enum."ElevDown", "Action2Trigger"=0, "WristPositions"=enum."AllDown", "SlowRng"=36.0, "TimeOut"=1.75, "GyroSens"=0.0, "DriveHeading"=225.0}, {"Action"=enum."StraightForward", "DriveEncCnts"=9500, "Accel?"=TRUE, "Decel?"=FALSE, "ElevEncCnts"=0, "Action2"=enum."ElevDown", "Action2Trigger"=0, "WristPositions"=enum."AllDown", "SlowRng"=0.0, "TimeOut"=10.0, "GyroSens"=0.006, "DriveHeading"=225.0}, {"Action"=enum."StraightForward", "DriveEncCnts"=7000, "Accel?"=FALSE, "Decel?"=TRUE, "ElevEncCnts"=0, "Action2"=enum."Intake", "Action2Trigger"=0, "WristPositions"=enum."AllDown", "SlowRng"=6000.0, "TimeOut"=10.0, "GyroSens"=0.00065, "DriveHeading"=225.0}, {"Action"=enum."Pause", "DriveEncCnts"=0, "Accel?"=FALSE, "Decel?"=FALSE, "ElevEncCnts"=0, "Action2"=enum."CubeCollect", "Action2Trigger"=0, "WristPositions"=enum."AllDown", "SlowRng"=0.0, "TimeOut"=0.5, "GyroSens"=0.0, "DriveHeading"=0.0}, {"Action"=enum."StraightBack", "DriveEncCnts"=-5000, "Accel?"=TRUE, "Decel?"=TRUE, "ElevEncCnts"=0, "Action2"=enum."Intake", "Action2Trigger"=0, "WristPositions"=enum."AllDown", "SlowRng"=-2000.0, "TimeOut"=10.0, "GyroSens"=0.00065, "DriveHeading"=225.0}, {"Action"=enum."Pause", "DriveEncCnts"=0, "Accel?"=FALSE, "Decel?"=FALSE, "ElevEncCnts"=17000, "Action2"=enum."ElevUp", "Action2Trigger"=0, "WristPositions"=enum."AllDown", "SlowRng"=0.0, "TimeOut"=1.0, "GyroSens"=0.0, "DriveHeading"=0.0}, {"Action"=enum."StraightForward", "DriveEncCnts"=7000, "Accel?"=TRUE, "Decel?"=TRUE, "ElevEncCnts"=0, "Action2"=enum."ShifterToggle", "Action2Trigger"=0, "WristPositions"=enum."AllDown", "SlowRng"=2000.0, "TimeOut"=1.5, "GyroSens"=0.00065, "DriveHeading"=225.0}, {"Action"=enum."Pause", "DriveEncCnts"=0, "Accel?"=FALSE, "Decel?"=FALSE, "ElevEncCnts"=0, "Action2"=enum."Release", "Action2Trigger"=0, "WristPositions"=enum."AllDown", "SlowRng"=0.0, "TimeOut"=1.5, "GyroSens"=0.0, "DriveHeading"=0.0}, {"Action"=enum."BackPivot", "DriveEncCnts"=0, "Accel?"=FALSE, "Decel?"=FALSE, "ElevEncCnts"=0, "Action2"=enum."", "Action2Trigger"=0, "WristPositions"=enum."AllDown", "SlowRng"=30.0, "TimeOut"=0.25, "GyroSens"=0.0, "DriveHeading"=247.5}, {"Action"=enum."Pause", "DriveEncCnts"=0, "Accel?"=FALSE, "Decel?"=FALSE, "ElevEncCnts"=0, "Action2"=enum."ElevDown", "Action2Trigger"=0, "WristPositions"=enum."AllDown", "SlowRng"=0.0, "TimeOut"=1.0, "GyroSens"=0.0, "DriveHeading"=0.0}, {"Action"=enum."StraightForward", "DriveEncCnts"=5000, "Accel?"=TRUE, "Decel?"=TRUE, "ElevEncCnts"=0, "Action2"=enum."Intake", "Action2Trigger"=0, "WristPositions"=enum."AllDown", "SlowRng"=2000.0, "TimeOut"=1.5, "GyroSens"=0.00065, "DriveHeading"=247.5}, {"Action"=enum."Pause", "DriveEncCnts"=0, "Accel?"=FALSE, "Decel?"=FALSE, "ElevEncCnts"=0, "Action2"=enum."CubeCollect", "Action2Trigger"=0, "WristPositions"=enum."AllDown", "SlowRng"=0.0, "TimeOut"=0.5, "GyroSens"=0.0, "DriveHeading"=0.0}, {"Action"=enum."StraightBack", "DriveEncCnts"=-10000, "Accel?"=FALSE, "Decel?"=TRUE, "ElevEncCnts"=0, "Action2"=enum."Intake", "Action2Trigger"=0, "WristPositions"=enum."AllDown", "SlowRng"=-7500.0, "TimeOut"=5.0, "GyroSens"=0.00065, "DriveHeading"=270.0}]] -> w10
    frame "DoNothing" {
    }
    frame "CrossLine", Default {
    }
    frame "CrossLineTime" {
    }
    frame "CenterSwitchL" {
    }
    frame "CenterSwitchR" {
    }
    frame "CenterSwitchSwitchL" {
    }
    frame "CenterSwitchSwitchR" {
    }
    frame "LeftSwitch" {
    }
    frame "RightSwitch" {
    }
    frame "LeftScale" {
    }
    frame "RightScale" {
    }
    frame "LeftCrossScale" {
    }
    frame "RightCrossScale" {
    }
    frame "LeftCrossCross" {
    }
    frame "RightCrossCross" {
    }
    frame "LeftCrossScaleScale" {
    }
    frame "RightCrossScaleScale" {
    }
    frame "LeftCrossScaleSwitch" {
    }
    frame "RightCrossScaleSwitch" {
    }
    frame "LeftScaleScale" {
    }
    frame "RightScaleScale" {
    }
    frame "LeftScaleSwitch" {
    }
    frame "RightScaleSwitch" {
    }
  }
  n3 = call-poly <vilib>:"NT Write Value.vi"("String"=w4, "Name"="AutonControl") -> ()  [unwired: 9 in, 1 out]
  n4 = while {
    stop <- FALSE stop-if-true
    n5 = call <vilib>:"WPI_DriverStationReport Robot Code State.vi"("Autonomous"=TRUE) -> ()  [unwired: 10 in, 1 out]
    n6 = Wait (ms)(milliseconds to wait=u32 20) -> ()  [unwired: 1 out]
  }
  n7 = call "DataLogging_v2.vi"("New Line?"=TRUE, "Name"="Auton Mode", "Variant In"=w4) -> ("error out"=w3:errorcluster)  [unwired: 7 in, 1 out]
  n8 = while {
    tunnel: w10 -> [w56]
    shift-right: [w93] -> _
    shift-left: 0 ("IndexOut") -> [w49]
    tunnel: w8 -> [w91]
    tunnel: w7 -> [w90]
    shift-right: [w81] -> _
    shift-left: w3 -> [w82]
    shift-right: [w45] -> _
    shift-left: TRUE -> [w79]
    shift-right: [w61] -> _
    shift-left: _ -> [w60]
    stop <- FALSE stop-if-true
    # "If new Action, log name"
    # "Log data if First Time, new Action, or 15 ms since the last Log"
    # "Data Logging"
    # "Manipulator Actions"
    # "Drive Actions"
    n9 = Array Size(array=w56) -> (size(s)=w55:i32)
    n10 = Decrement(x=w55) -> (x-1=w54:i32)
    n11 = Decrement(x=w49) -> (x-1=w52:i32)
    n12 = Greater?(x=w49, y=w54) -> (0:w53:bool)
    n13 = Select(t=w52, s=w53, f=w49) -> (s? t:f=w48:i32)
    n14 = Index Array(array=w56, index=w48) -> (element=w71:T6)
    n15 = Unbundle By Name(w71) -> ("GyroSens"=w40:dbl, "DriveHeading"=w42:dbl, "Accel?"=w89:bool, "Decel?"=w88:bool, "SlowRng"=w67:dbl, "DriveEncCnts"=w76:i32, "TimeOut"=w50:dbl, "Action"=w39:T3)
    n16 = Unbundle By Name(w71) -> ("Action2Trigger"=w70:i32, "Action2"=w38:T3, "WristPositions"=w69:T4, "ElevEncCnts"=w68:i32, "TimeOut"=w47:dbl)
    n17 = Tick Count (ms)() -> (millisecond timer value=w64:u32)
    n18 = Subtract(x=w64, y=w60) -> (x-y=w63:u32)
    n19 = First Call?() -> (First Call?: T/F=w58:bool)
    n20 = call "Is Value Changed.vim"("value"=w48) -> ("changed or first call?"=w41:bool)
    n21 = Greater Or Equal?(x=w63, y=u32 15) -> (x >= y?=w59:bool)
    n22 = case shown="\"StraightForward\"" w39 {
      tunnel: [w113 w141 w174 w195 w214 w233 w243 w250 w254] -> w93
      tunnel: w48 -> [w114 w126 w159 w191 w210 w229 w240 w251 w253]
      tunnel: [_ w144 w177 w194 w213 w232 w242 w249 w255] -> w83
      tunnel: [_ w140 w173 w193 w212 w231 w242 w249 w255] -> w84
      tunnel: w76 -> [_ w132 w165 _ _ _ _ _ _]
      tunnel: w89 -> [_ w119 w152 _ _ _ _ _ _]
      tunnel: w88 -> [_ w116 w149 _ _ _ _ _ _]
      tunnel: w91 -> [_ w137 w170 _ _ _ _ _ _]
      tunnel: w90 -> [_ w115 w148 _ _ _ _ _ _]
      tunnel: [_ w118 w151 w184 w203 w222 _ _ _] -> w87
      tunnel: [_ w122 w155 w183 w202 w221 _ _ _] -> w86
      tunnel: [_ w134 w167 _ _ _ _ _ _] -> w74
      tunnel: [_ w131 w164 _ _ _ _ _ _] -> w85
      tunnel: [_ w130 w163 _ _ _ _ _ _] -> w73
      tunnel: w67 -> [_ w128 w161 w192 w211 w230 _ _ _]
      tunnel: w50 -> [_ w125 w158 w188 w207 w226 w241 w246 _]
      tunnel: w40 -> [_ w127 w160 _ _ _ _ _ _]
      tunnel: w42 -> [_ w122 w155 w183 w202 w221 _ _ _]
      tunnel: w41 -> [_ w117 w150 w182 w201 w220 w238 w244 _]
      frame "Initialize" {
        w95 = FALSE ("MostDown")
        # "Initialize sensors and solenoid positions.\nDon't move on until reset of Drive Encoders and Gyro are confirmed"
        n23 = call "Wrist.vi"("Up"=w95, "Down"=w95) -> ()  [unwired: 6 in]
        n24 = call "Shifter.vi"("Shift?"=FALSE) -> ()  [unwired: 3 in]
        n25 = call "Gripper.vi"("Grip"=FALSE) -> ()  [unwired: 3 in]
        n26 = call "ElevEnc.vi"("Reset?"=TRUE) -> ()  [unwired: 10 in, 1 out]
        n27 = call "GyroActions.vi"("Zero"=TRUE) -> ("Fused Heading"=w110:dbl)  [unwired: 9 in, 1 out]
        n28 = call "ElevShifter.vi"("Shift?"=FALSE) -> ()  [unwired: 8 in, 1 out]
        n29 = call "DriveEnc.vi"("Reset?"=TRUE) -> ("RightEncder"=w105:dbl)  [unwired: 9 in, 1 out]
        n30 = Greater?(x=w110, y=359.5 ("upper limit")) -> (0:w108:bool)
        n31 = Less?(x=w110, y=0.5 ("lower limit")) -> (x < y?=w111:bool)
        n32 = Or(x=w108, y=w111) -> (x .or. y?=w102:bool)
        n33 = Greater?(x=w105, y=-20.0) -> (0:w101:bool)
        n34 = Less?(x=w105, y=20.0) -> (x < y?=w100:bool)
        n35 = Compound Arithmetic op=AND(w102, w101, w100) -> (w94:bool)
        n36 = call "IncrementIndex.vi"("Increment?"=w94, "IndexIn"=w114) -> ("IndexOut"=w113:i32)  [unwired: 9 in]
      }
      frame "StraightForward" {
        w139 = -1.0  # MaxPwr
        w138 = 0.15  # MinPwr
        w120 = 0.25  # ErrorRange
        # "Hold initial value"
        # "When finished, only stop motors if Decel? is true.\nOtherwise, move into next action without stopping motors.\nUsed when moving into another Drive action"
        # "Time out if action runs too long"
        # "Negative\n= Forward"
        n37 = call "GyroActions.vi"() -> ("Fused Heading"=w118:dbl)  [unwired: 10 in, 1 out]
        n38 = call "Wait.vi"("Target Time (s)"=w125, "First Time?"=w117) -> ("Completed"=w124:bool)  [unwired: 8 in, 1 out]
        n39 = call "DriveEnc.vi"() -> ("RightEncder"=w134:dbl)  [unwired: 10 in, 1 out]
        n40 = Bundle By Name(cluster=w137, "Range"=w120, "GyroSens"=w127, "Target"=w122, "Heading"=w118) -> (w136:T2)
        n41 = feedback #1() -> (w133:dbl)  [unwired: 1 in]
        n42 = Select(t=w134, s=w117, f=w133) -> (s? t:f=w130:dbl)
        n43 = feedback-in #1(w130) -> ()
        n44 = Add(x=w132, y=w130) -> (x+y=w131:dbl)
        n45 = Greater Or Equal?(x=w134, y=w131) -> (x >= y?=w123:bool)
        n46 = Or(x=w123, y=w124) -> (x .or. y?=w121:bool)
        n47 = Bundle By Name(cluster=w115, "SlowRng"=w128, "CurrCounts"=w134, "TrgtCounts"=w131) -> (w135:T1)
        n48 = call "DriveStraight.vi"("EncData"=w135, "FirstTime?"=w117, "GyroData"=w136, "Decel?"=w116, "Accel?"=w119, "MinPwr"=w138, "MaxPwr"=w139) -> ("RightOut"=w143:dbl, "LeftOut"=w142:dbl)  [unwired: 3 in]
        n49 = And(x=w116, y=w121) -> (x .and. y?=w129:bool)
        n50 = call "IncrementIndex.vi"("Increment?"=w121, "IndexIn"=w126) -> ("IndexOut"=w141:i32)  [unwired: 9 in]
        n51 = case shown="True" w129 {
          tunnel: [w146 w147] -> w144
          tunnel: w142 -> [w146 _]
          tunnel: w143 -> [w145 _]
          tunnel: [w145 w147] -> w140
          frame False {
          }
          frame True {
            w147 = 0.0 ("Left")
          }
        }
      }
      frame "StraightBack" {
        w172 = 1.0  # MaxPwr
        w171 = 0.15  # MinPwr
        w153 = 0.25  # ErrorRange
        # "Hold initial value"
        # "When finished, only stop motors if Decel? is true.\nOtherwise, move into next action without stopping motors.\nUsed when moving into another Drive action"
        # "Time out if action runs too long"
        # "Positive\n= Back"
        n52 = call "GyroActions.vi"() -> ("Fused Heading"=w151:dbl)  [unwired: 10 in, 1 out]
        n53 = call "Wait.vi"("Target Time (s)"=w158, "First Time?"=w150) -> ("Completed"=w157:bool)  [unwired: 8 in, 1 out]
        n54 = call "DriveEnc.vi"() -> ("RightEncder"=w167:dbl)  [unwired: 10 in, 1 out]
        n55 = Bundle By Name(cluster=w170, "Range"=w153, "GyroSens"=w160, "Target"=w155, "Heading"=w151) -> (w169:T2)
        n56 = feedback #2() -> (w166:dbl)  [unwired: 1 in]
        n57 = Select(t=w167, s=w150, f=w166) -> (s? t:f=w163:dbl)
        n58 = feedback-in #2(w163) -> ()
        n59 = Add(x=w165, y=w163) -> (x+y=w164:dbl)
        n60 = Less Or Equal?(x=w167, y=w164) -> (x <= y?=w156:bool)
        n61 = Or(x=w156, y=w157) -> (x .or. y?=w154:bool)
        n62 = Bundle By Name(cluster=w148, "SlowRng"=w161, "CurrCounts"=w167, "TrgtCounts"=w164) -> (w168:T1)
        n63 = call "DriveStraight.vi"("EncData"=w168, "FirstTime?"=w150, "GyroData"=w169, "Decel?"=w149, "Accel?"=w152, "MinPwr"=w171, "MaxPwr"=w172) -> ("RightOut"=w176:dbl, "LeftOut"=w175:dbl)  [unwired: 3 in]
        n64 = And(x=w149, y=w154) -> (x .and. y?=w162:bool)
        n65 = call "IncrementIndex.vi"("Increment?"=w154, "IndexIn"=w159) -> ("IndexOut"=w174:i32)  [unwired: 9 in]
        n66 = case shown="True" w162 {
          tunnel: [w179 w180] -> w177
          tunnel: w175 -> [w179 _]
          tunnel: w176 -> [w178 _]
          tunnel: [w178 w180] -> w173
          frame False {
          }
          frame True {
            w180 = 0.0 ("Left")
          }
        }
      }
      frame "GeneralTurn" {
        w197 = 1.0  # Max Power
        w198 = 0.25  # Error Range
        w199 = 0.5  # Min Power
        # "Hold initial Distance and Direction for current turn Action"
        n67 = call "Wait.vi"("Target Time (s)"=w188, "First Time?"=w182) -> ("Completed"=w190:bool)  [unwired: 8 in, 1 out]
        n68 = call "GyroActions.vi"() -> ("Fused Heading"=w184:dbl)  [unwired: 10 in, 1 out]
        n69 = call "HeadingCalc.vi"("Target"=w183, "Current"=w184) -> ("Dis&Dir"=w187:dbl)  [unwired: 9 in]
        n70 = feedback #3() -> (w186:dbl)  [unwired: 1 in]
        n71 = Select(t=w187, s=w182, f=w186) -> (s? t:f=w185:dbl)
        n72 = feedback-in #3(w185) -> ()
        n73 = call "TurnSmooth.vi"("Pivot?"=FALSE ("Pivot"), "MinPower"=w199, "FirstTime?"=w182, "ErrorRange"=w198, "CurrentPosition"=w184, "Dir&Deg"=w185, "SlowRange"=w192, "MaxPower"=w197) -> ("Done"=w189:bool, "RightMotorPower"=w193:dbl, "LeftMotorPower"=w194:dbl)  [unwired: 1 out]
        n74 = Or(x=w189, y=w190) -> (x .or. y?=w181:bool)
        n75 = call "IncrementIndex.vi"("Increment?"=w181, "IndexIn"=w191) -> ("IndexOut"=w195:i32)  [unwired: 9 in]
      }
      frame "ForwardPivot" {
        w216 = 1.0  # Max Power
        w217 = 0.5  # Error Range
        w218 = 0.5  # Min Power
        # "Hold initial Distance and Direction for current turn Action"
        n76 = call "Wait.vi"("Target Time (s)"=w207, "First Time?"=w201) -> ("Completed"=w209:bool)  [unwired: 8 in, 1 out]
        n77 = call "GyroActions.vi"() -> ("Fused Heading"=w203:dbl)  [unwired: 10 in, 1 out]
        n78 = call "HeadingCalc.vi"("Target"=w202, "Current"=w203) -> ("Dis&Dir"=w206:dbl)  [unwired: 9 in]
        n79 = feedback #4() -> (w205:dbl)  [unwired: 1 in]
        n80 = Select(t=w206, s=w201, f=w205) -> (s? t:f=w204:dbl)
        n81 = feedback-in #4(w204) -> ()
        n82 = call "TurnSmooth.vi"("Pivot?"=TRUE ("Pivot"), "MinPower"=w218, "FirstTime?"=w201, "ErrorRange"=w217, "CurrentPosition"=w203, "Dir&Deg"=w204, "SlowRange"=w211, "MaxPower"=w216) -> ("Done"=w208:bool, "RightMotorPower"=w212:dbl, "LeftMotorPower"=w213:dbl)  [unwired: 1 out]
        n83 = Or(x=w208, y=w209) -> (x .or. y?=w200:bool)
        n84 = call "IncrementIndex.vi"("Increment?"=w200, "IndexIn"=w210) -> ("IndexOut"=w214:i32)  [unwired: 9 in]
      }
      frame "BackPivot" {
        w235 = -1.0  # Max Power
        w236 = 0.5  # Error Range
        w237 = 0.5  # Min Power
        # "Hold initial Distance and Direction for current turn Action"
        n85 = call "Wait.vi"("Target Time (s)"=w226, "First Time?"=w220) -> ("Completed"=w228:bool)  [unwired: 8 in, 1 out]
        n86 = call "GyroActions.vi"() -> ("Fused Heading"=w222:dbl)  [unwired: 10 in, 1 out]
        n87 = call "HeadingCalc.vi"("Target"=w221, "Current"=w222) -> ("Dis&Dir"=w225:dbl)  [unwired: 9 in]
        n88 = feedback #5() -> (w224:dbl)  [unwired: 1 in]
        n89 = Select(t=w225, s=w220, f=w224) -> (s? t:f=w223:dbl)
        n90 = feedback-in #5(w223) -> ()
        n91 = call "TurnSmooth.vi"("Pivot?"=TRUE ("Pivot"), "MinPower"=w237, "FirstTime?"=w220, "ErrorRange"=w236, "CurrentPosition"=w222, "Dir&Deg"=w223, "SlowRange"=w230, "MaxPower"=w235) -> ("Done"=w227:bool, "RightMotorPower"=w231:dbl, "LeftMotorPower"=w232:dbl)  [unwired: 1 out]
        n92 = Or(x=w227, y=w228) -> (x .or. y?=w219:bool)
        n93 = call "IncrementIndex.vi"("Increment?"=w219, "IndexIn"=w229) -> ("IndexOut"=w233:i32)  [unwired: 9 in]
      }
      frame "Pause" {
        w242 = 0.0 ("Left Motor Power")
        n94 = call "Wait.vi"("Target Time (s)"=w241, "First Time?"=w238) -> ("Completed"=w239:bool)  [unwired: 8 in, 1 out]
        n95 = call "IncrementIndex.vi"("Increment?"=w239, "IndexIn"=w240) -> ("IndexOut"=w243:i32)  [unwired: 9 in]
      }
      frame "StraightForwardTime" {
        # "A drive forward based on time in case encoders fail and no time to fix"
        n96 = call "Wait.vi"("Target Time (s)"=w246, "First Time?"=w244) -> ("Completed"=w245:bool)  [unwired: 8 in, 1 out]
        n97 = call "IncrementIndex.vi"("Increment?"=w245, "IndexIn"=w251) -> ("IndexOut"=w250:i32)  [unwired: 9 in]
        n98 = Select(t=0.0, s=w245, f=1.0) -> (s? t:f=w249:dbl)
      }
      frame "Stop", Default {
        w255 = 0.0 ("Left Motor Power")
        n99 = call "IncrementIndex.vi"("Increment?"=TRUE, "IndexIn"=w253) -> ("IndexOut"=w254:i32)  [unwired: 9 in]
      }
    }
    n100 = Compound Arithmetic op=OR(w41, w58, w59) -> (w57:bool)
    n101 = call "Is Value Changed.vim"("value"=w38) -> ("changed or first call?"=w37:bool)
    n102 = Format Into String(w38) -> (resulting string=w80:string)  [unwired: 3 in, 1 out]
    n103 = Empty String/Path?(string/path=w80) -> (empty?=w72:bool)
    n104 = Select(t=FALSE, s=w37, f=w79) -> (s? t:f=w51:bool)
    n105 = call "Action2Trigger.vi"("NewAction?"=w37, "TriggerCount"=w70, "Enc Initial"=w73, "Current"=w74) -> ("Triggered?"=w75:bool)  [unwired: 7 in]
    n106 = Compound Arithmetic op=AND(w75, invert w72, invert w51) -> (w77:bool)
    n107 = case shown="True" w77 {
      tunnel: [w305 w313] -> w45
      tunnel: w38 -> [_ w316]
      tunnel: [_ w315] -> w66
      tunnel: [_ w314] -> w65
      tunnel: w69 -> [_ w312]
      tunnel: w68 -> [_ w311]
      tunnel: w37 -> [_ w310]
      tunnel: w51 -> [w305 _]
      tunnel: w47 -> [_ w309]
      tunnel: [_ w308] -> w46
      tunnel: [_ w307] -> w44
      tunnel: [_ w306] -> w43
      frame False {
      }
      frame True {
        n108 = case shown="\"Wrist\"" w316 {
          tunnel: [_ _ _ -0.85 ("Left Motor Power") 0.6 ("Left Motor Power") _ _ _ _ _] -> w315
          tunnel: [_ 0.4 ("Left Motor Power") 1.0 ("Left Motor Power") _ _ _ _ _ -0.7 ("Left Motor Power") -1.0 ("Left Motor Power")] -> w314
          tunnel: [_ w320 w327 w338 w344 TRUE ("Grip") w353 w354 w356 _] -> w313
          tunnel: w312 -> [_ _ _ _ _ w350 _ _ _ _]
          tunnel: w311 -> [_ _ _ w339 w347 _ _ _ _ _]
          tunnel: w310 -> [_ w321 w333 _ _ _ _ _ w358 _]
          tunnel: w309 -> [_ w319 _ _ _ _ _ _ w357 _]
          tunnel: [_ _ _ _ TRUE ("Shift?") _ _ w354 _ _] -> w308
          tunnel: [_ _ _ _ TRUE ("Grip") _ w353 _ TRUE ("Grip") _] -> w307
          tunnel: [_ _ _ w335 w342 _ _ _ _ _] -> w306
          frame "Initialize", Default {
            # "Nothing to initialize; it just sets all Manipulator motors and solenoids to their default values"
          }
          frame "Release" {
            # "Run Intake at low speed for a Time"
            n109 = Tick Count (ms)() -> (millisecond timer value=w324:u32)
            n110 = Multiply(x=1000.0, y=w319) -> (x*y=w317:dbl)
            n111 = feedback #6() -> (w325:u32)  [unwired: 1 in]
            n112 = Select(t=w324, s=w321, f=w325) -> (s? t:f=w323:u32)
            n113 = feedback-in #6(w323) -> ()
            n114 = Subtract(x=w324, y=w323) -> (x-y=w322:u32)
            n115 = Greater Or Equal?(x=w322, y=w317) -> (x >= y?=w320:bool)
          }
          frame "Shoot" {
            # "Run Intake at high speed for a Time"
            n116 = Tick Count (ms)() -> (millisecond timer value=w331:u32)
            n117 = feedback #7() -> (w332:u32)  [unwired: 1 in]
            n118 = Select(t=w331, s=w333, f=w332) -> (s? t:f=w330:u32)
            n119 = feedback-in #7(w330) -> ()
            n120 = Subtract(x=w331, y=w330) -> (x-y=w329:u32)
            n121 = Greater Or Equal?(x=w329, y=u32 2000) -> (x >= y?=w327:bool)
          }
          frame "ElevUp" {
            # "Raise Elevator"
            n122 = call "ElevEnc.vi"() -> ("ElevEnc"=w335:dbl)  [unwired: 11 in]
            n123 = Greater Or Equal?(x=w335, y=w339) -> (x >= y?=w337:bool)
            n124 = call "ElevLimits.vi"() -> ("UpLimit"=w336:bool)  [unwired: 9 in, 2 out]
            n125 = Or(x=w336, y=w337) -> (x .or. y?=w338:bool)
          }
          frame "ElevDown" {
            # "Lower Elevator"
            n126 = call "ElevEnc.vi"() -> ("ElevEnc"=w342:dbl)  [unwired: 11 in]
            n127 = Less Or Equal?(x=w342, y=w347) -> (x <= y?=w346:bool)
            n128 = call "ElevLimits.vi"() -> ("BotLimit"=w345:bool)  [unwired: 9 in, 2 out]
            n129 = Or(x=w345, y=w346) -> (x .or. y?=w344:bool)
          }
          frame "Wrist" {
            # "Put Wrist in specified position"
            n130 = case shown="\"AllDown\", Default" w350 {
              frame "AllUp" {
                n131 = call "Wrist.vi"("Down"=TRUE ("AllDown")) -> ()  [unwired: 7 in]
              }
              frame "AllDown", Default {
                n132 = call "Wrist.vi"("Up"=TRUE ("AllUp")) -> ()  [unwired: 7 in]
              }
            }
          }
          frame "GripperToggle" {
            w353 = TRUE ("Grip")
            # "Toggle Gripper open/closed"
          }
          frame "ShifterToggle" {
            w354 = TRUE ("Shift?")
            # "Toggle Elevator Shifter"
          }
          frame "CubeCollect" {
            # "Close Gripper and run Intake to grab cube"
            n133 = call "Wait.vi"("Target Time (s)"=w357, "First Time?"=w358) -> ("Completed"=w356:bool)  [unwired: 8 in, 1 out]
          }
          frame "Intake" {
            # "Run Intake to pull the cube in farther"
          }
        }
      }
    }
    n134 = case shown="True" w57 {
      tunnel: w87 -> [_ w278]
      tunnel: w86 -> [_ w280]
      tunnel: w85 -> [_ w270]
      tunnel: w84 -> [_ w260]
      tunnel: w83 -> [_ w262]
      tunnel: w82 -> [w257 w295]
      tunnel: [w257 w289] -> w81
      tunnel: w41 -> [_ w293]
      tunnel: w39 -> [_ w292]
      tunnel: w66 -> [_ w266]
      tunnel: w65 -> [_ w268]
      tunnel: w58 -> [_ w291]
      tunnel: [w256 w290] -> w61
      tunnel: w60 -> [w256 _]
      tunnel: w43 -> [_ w264]
      frame False {
      }
      frame True {
        n135 = Or(x=w293, y=w291) -> (x .or. y?=w294:bool)
        n136 = case shown="True" w294 {
          tunnel: w292 -> [_ w302]
          tunnel: [w299 w303] -> w277
          tunnel: w295 -> [w298 w304]
          frame False {
            n137 = call "DataLogging_v2.vi"("Name"="", "error in (no error)"=w298, "Variant In"="\t") -> ("error out"=w299:errorcluster)  [unwired: 7 in, 1 out]
          }
          frame True {
            w301 = TRUE ("New Line?")
            n138 = call "DataLogging_v2.vi"("Tab?"=w301, "New Line?"=w301, "Name"="Action", "error in (no error)"=w304, "Variant In"=w302) -> ("error out"=w303:errorcluster)  [unwired: 5 in, 1 out]
          }
        }
        n139 = call "DataLogging_v2.vi"("Name"="Gyro Current", "error in (no error)"=w277, "Variant In"=w278) -> ("error out"=w279:errorcluster)  [unwired: 7 in, 1 out]
        n140 = call "DataLogging_v2.vi"("Name"="Gyro Target", "error in (no error)"=w279, "Variant In"=w280) -> ("error out"=w281:errorcluster)  [unwired: 7 in, 1 out]
        n141 = call "DriveEnc.vi"() -> ("RightEncder"=w273:dbl, "LeftEncoder"=w272:dbl)  [unwired: 10 in]
        n142 = call "DataLogging_v2.vi"("Name"="LeftEnc", "error in (no error)"=w281, "Variant In"=w272) -> ("error out"=w282:errorcluster)  [unwired: 7 in, 1 out]
        n143 = call "DataLogging_v2.vi"("Name"="RightEnc", "error in (no error)"=w282, "Variant In"=w273) -> ("error out"=w283:errorcluster)  [unwired: 7 in, 1 out]
        n144 = call "DataLogging_v2.vi"("Name"="Enc Target", "error in (no error)"=w283, "Variant In"=w270) -> ("error out"=w284:errorcluster)  [unwired: 7 in, 1 out]
        n145 = call "DataLogging_v2.vi"("Name"="IntakePwr", "error in (no error)"=w284, "Variant In"=w268) -> ("error out"=w285:errorcluster)  [unwired: 7 in, 1 out]
        n146 = call "DataLogging_v2.vi"("Name"="ElevPwr", "error in (no error)"=w285, "Variant In"=w266) -> ("error out"=w286:errorcluster)  [unwired: 7 in, 1 out]
        n147 = call "DataLogging_v2.vi"("Name"="ElevEnc", "error in (no error)"=w286, "Variant In"=w264) -> ("error out"=w287:errorcluster)  [unwired: 7 in, 1 out]
        n148 = call "DataLogging_v2.vi"("Name"="DriveLeftPwr", "error in (no error)"=w287, "Variant In"=w262) -> ("error out"=w288:errorcluster)  [unwired: 7 in, 1 out]
        n149 = call "DataLogging_v2.vi"("New Line?"=TRUE, "Name"="DriveRightPwr", "error in (no error)"=w288, "Variant In"=w260) -> ("error out"=w289:errorcluster)  [unwired: 6 in, 1 out]
        n150 = Tick Count (ms)() -> (millisecond timer value=w290:u32)
      }
    }
    n151 = call "Intake.vi"("Power"=w65) -> ()  [unwired: 11 in]
    n152 = call "ElevShifter.vi"("Shift?"=w46) -> ()  [unwired: 8 in, 1 out]
    n153 = call "Gripper.vi"("Grip"=w44) -> ()  [unwired: 3 in]
    n154 = call "Elevator.vi"("Power"=w66) -> ()  [unwired: 11 in]
    n155 = call "Drive_4CANTank.vi"("RightMotor"=w84, "LeftMotor"=w83) -> ()  [unwired: 10 in]
  }
